vi "Main UI (ext control).vi"(0 "Serial port":refnum<visa-resource-name>="COM1", 1 "Command":T2, 5 "Data rate (Hz)":dbl=100.0, 7 "Max. num. sensors (override)":u8=64 max=64, 9 "Wait for HW trigger":bool, 11 "Finite samples":bool=TRUE, 12 "N samples":u32=1000, 14 "Error in":errorcluster) -> (4 "P data (mode 0)":T8[](array[typedef]), 15 "Error out":errorcluster)   [LabVIEW 2015]
doc: "User interface for 64 pressure multiplexer system designed by Paul Nathan, 02/2016"
uses:
  Ctls/System status.ctl
  Ctls/Environmental state values.ctl
  Ctls/Inertial state values.ctl
  Ctls/AccelGyro constants.ctl
  Ctls/Pressure sensor constants.ctl
  Ctls/Cmd list.ctl
  Ctls/Data values, Mode 0 (for datalog).ctl
  Ctls/Cmd str.ctl
  Ctls/All state values (for datalog).ctl
  Ctls/Data values, Mode 1 (for datalog).ctl
  Globals/PressureMultiplexer global.vi
panel:
  in  "Main tabs":T1(tab)
  in  "Env. period (ms)":i32=1000 min=0
  out "ACK 8":bool caption="ACK"
  out "ACK 7":bool caption="ACK"
  out "ACK 6":bool caption="ACK"
  out "AccelGyro constants":T3={"gyrRange"=125.0, "accRange"=2.0, "gx offset"=0.0, "gy offset"=0.0, "gz offset"=0.0, "ax offset"=0.0, "ay offset"=0.0, "az offset"=0.0, "axyz scale"=1.0} {"axyz scale" format="%#_4f"; "az offset" format="%#_4f"; "ay offset" format="%#_4f"; "ax offset" format="%#_4f"; "gz offset" format="%#_4f"; "gy offset" format="%#_4f"; "gx offset" format="%#_4f"; "gyrRange" format="%#_4f"; "accRange" format="%#_4f"}
  out "Faulty sensors":i32[](array[numeric])
  out "ACK 5":bool caption="ACK"
  out "Active sensors":i32[](array[numeric])
  out "ACK 4":bool caption="ACK"
  in  "Gyro. rate (Hz)":u8(ring) items=["6.25", "12.5", "25", "50", "100", "200", "400", "800", "1600", "3200"]
  in  "Gyro. range (dps)":u8(ring) items=["+/- 125", "+/- 250", "+/- 500", "+/- 1000", "+/- 2000"]
  in  "Accel. rate (Hz)":u8(ring)=1 items=["3.125", "6.25", "12.5", "25", "50", "100", "200", "400", "800", "1600"]
  in  "Accel. range (g)":u8(ring) items=["+/- 2", "+/- 4", "+/- 8", "+/- 16"]
  out "Inertial state values":T4 {"w_z (dps)" format="%#_4f"; "a_y (g)" format="%#_4f"; "a_z (g)" format="%#_4f"; "w_y (dps)" format="%#_4f"; "a_x (g)" format="%#_4f"; "Sensor temp. (degC)" format="%#.2f"; "w_x (dps)" format="%#_4f"}
  out "Environmental state values":T5 {"Dew point (degC)" format="%#.2f"; "Density (kg/m^3)" format="%#.3f"; "Pressure alt. (m)" format="%#.2f"; "Density alt. (m)" format="%#.2f"; "Rel. Humidity (%)" format="%#.2f"; "P_atmos (Pa)" format="%#_6f"; "Sensor temp. (degC)" format="%#.2f"; "Thermistor (degC)" format="%#.2f"}
  out "System status":T6
  out "ACK 3":bool caption="ACK"
  out "ACK 1":bool caption="ACK"
  in  "Data mode":u8(ring) items=["P", "P & T"]
  out "ACK 2":bool caption="ACK"
  out "Main Power":bool
  out "L_data (bytes)":u16
  out "Serial no.":u16 format="%04x"
  out "Active pressure sensor constants":T7[](array[typedef])
  out "Streaming":bool
  out "Clock drift":bool
  in  "Display rate (Hz)":dbl=100.0 min=0.0
  out "Sensor temperatures time trace (Mode \"P & T\" only)":sgl[][](graph)
  out "Pressures time trace":sgl[][](graph)
  in  "Stop streaming":bool
  out "Stale samples flag":u8[][](graph)
  out "Samples acquired":u32
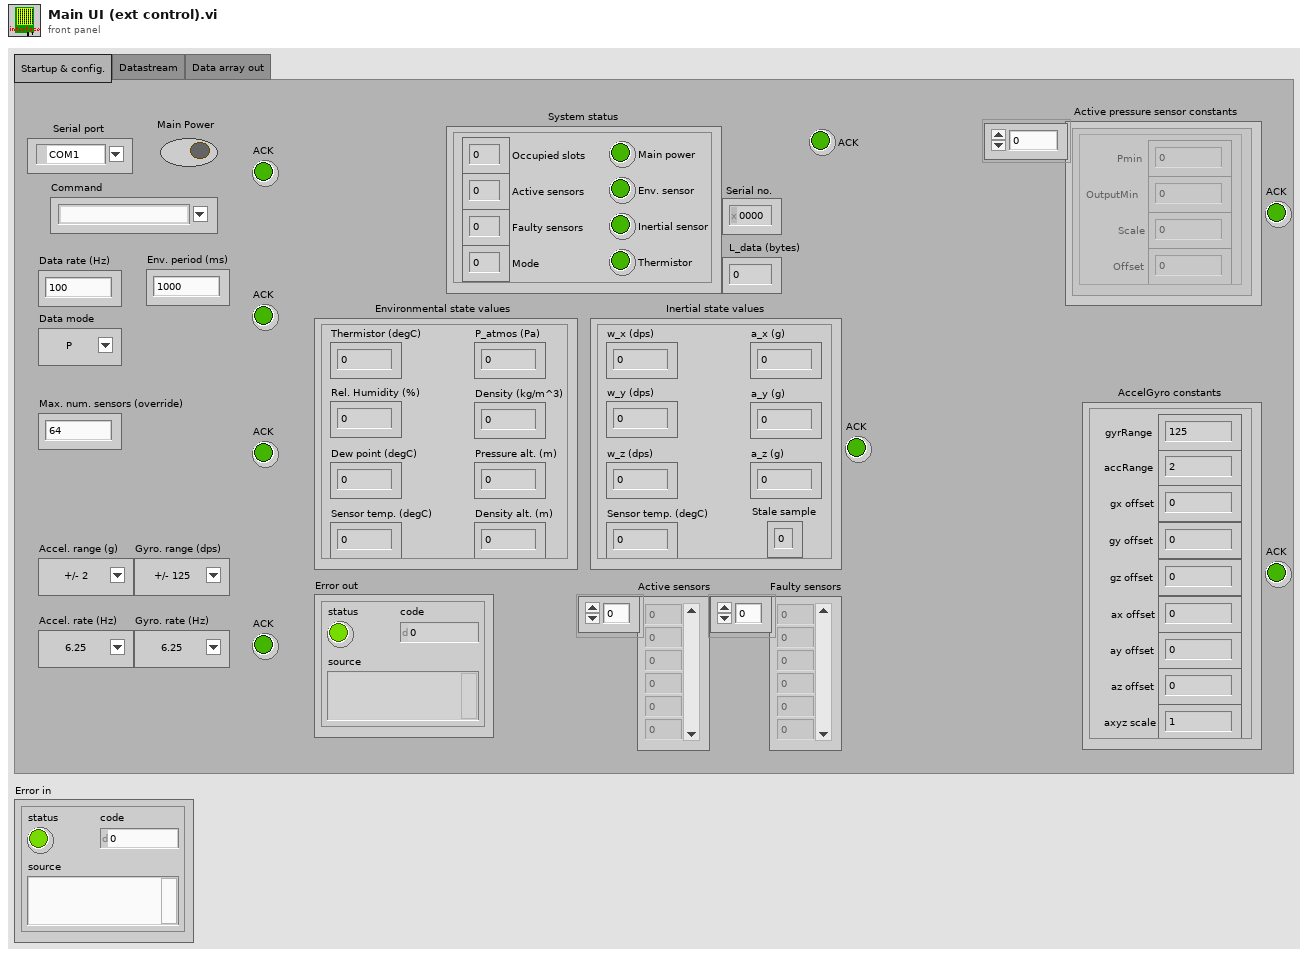
[diagram p1: front panel]
types:
  T1 = enum32{"Startup & config.", "Datastream", "Data array out"}
  T2 = typedef "Cmd list.ctl" = string
  T3 = typedef "AccelGyro constants.ctl" = cluster{"gyrRange":sgl, "accRange":sgl, "gx offset":sgl, "gy offset":sgl, "gz offset":sgl, "ax offset":sgl, "ay offset":sgl, "az offset":sgl, "axyz scale":sgl}
  T4 = typedef "Inertial state values.ctl" = cluster{"w_x (dps)":sgl, "w_y (dps)":sgl, "w_z (dps)":sgl, "a_x (g)":sgl, "a_y (g)":sgl, "a_z (g)":sgl, "Stale sample":u8, "Sensor temp. (degC)":sgl}
  T5 = typedef "Environmental state values.ctl" = cluster{"Thermistor (degC)":sgl, "Sensor temp. (degC)":sgl, "P_atmos (Pa)":sgl, "Rel. Humidity (%)":sgl, "Density (kg/m^3)":sgl, "Dew point (degC)":sgl, "Pressure alt. (m)":sgl, "Density alt. (m)":sgl}
  T6 = typedef "System status.ctl" = cluster{"Main power":bool, "Occupied slots":u8, "Active sensors":u8, "Faulty sensors":u8, "Env. sensor":bool, "Inertial sensor":bool, "Thermistor":bool, "Mode":u8}
  T7 = typedef "Pressure sensor constants.ctl" = cluster{"Pmin":sgl, "OutputMin":sgl, "Scale":sgl, "Offset":sgl}
  T8 = typedef "Data values, Mode 0 (for datalog).ctl" = cluster{"Time Stamp":timestamp, "dt (us)":sgl, "dt_warn":u8, "Pressures":sgl[], "Statuses":u8[]}
  T9 = typedef "All state values (for datalog).ctl" = cluster{"Time Stamp":timestamp, "dt (ms)":i32, "Environmental state values":T5, "Inertial state values":T4}
  T10 = typedef "Cmd str.ctl" = string
  T11 = typedef "Data values, Mode 1 (for datalog).ctl" = cluster{"Time Stamp":timestamp, "dt (us)":sgl, "dt_warn":u8, "Pressures":sgl[], "Die temps.":sgl[], "Statuses":u8[]}
  T12 = enum8{"Enabled", "Disabled", "Disabled and Grayed Out"}
  T13 = typedef "EEPROM page.ctl" = cluster{"Pmin (Pa)":sgl, "Pmax (Pa)":sgl, "maxCount":u16, "minCount":u16, "Poffset (Pa)":sgl}
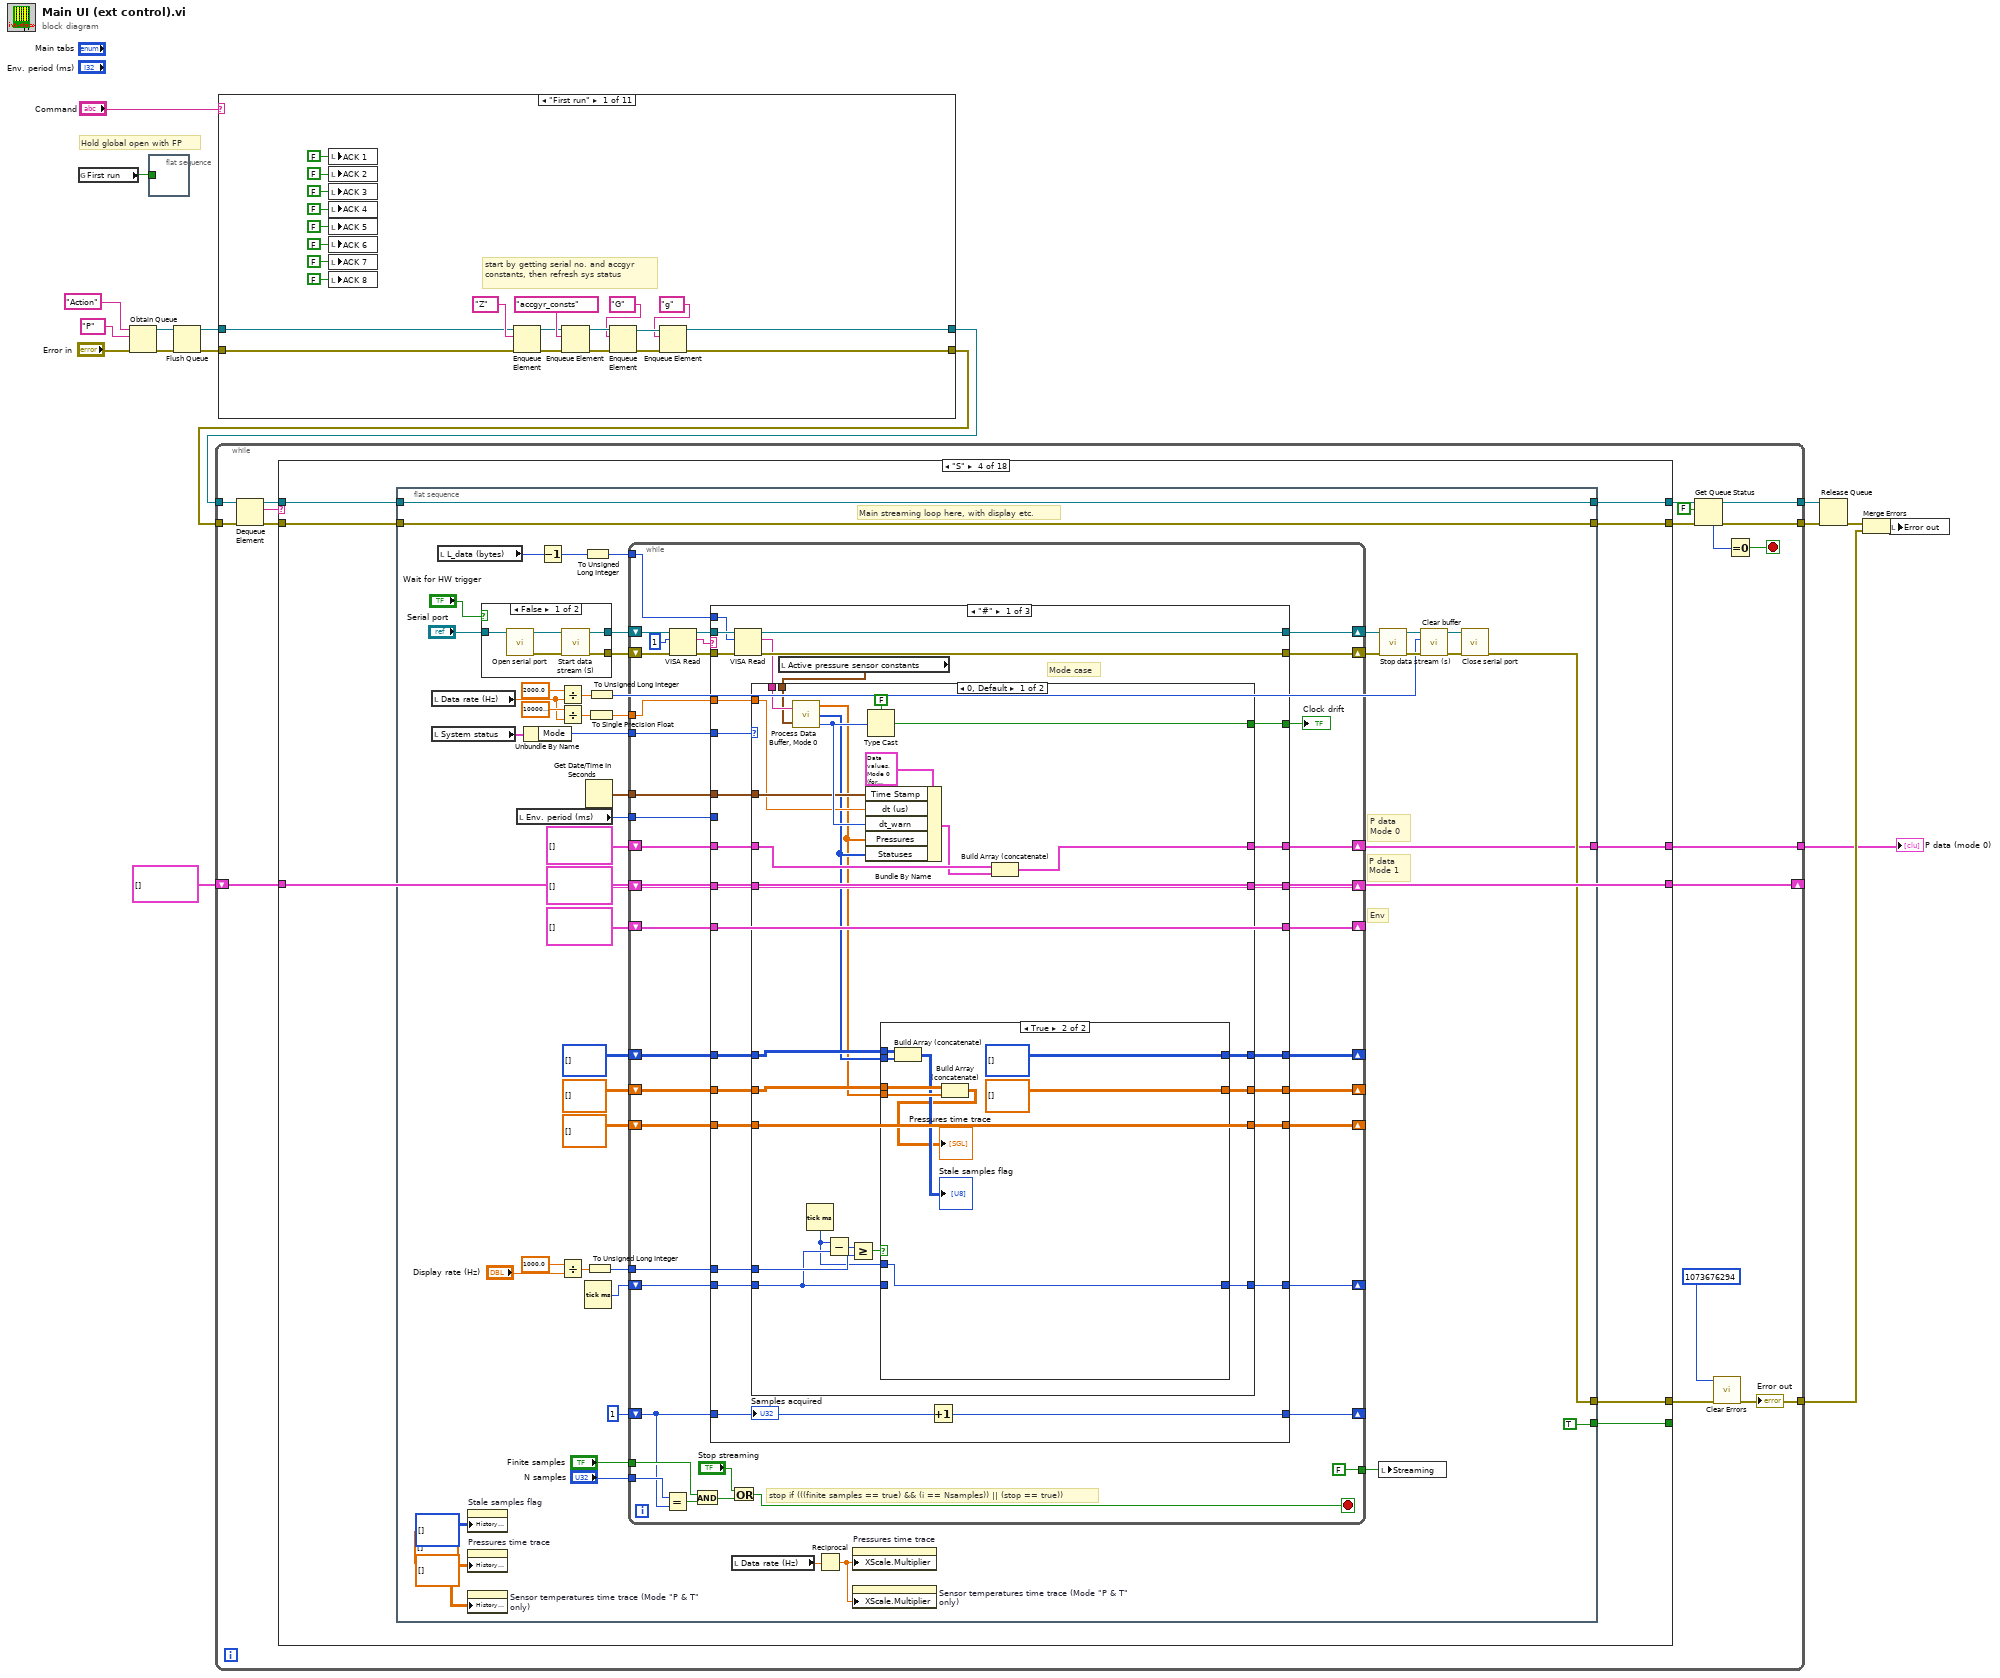
[diagram p0: block diagram]
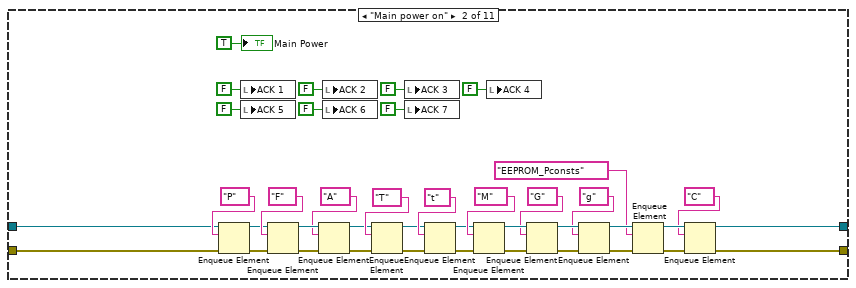
[diagram p2: hidden frame]
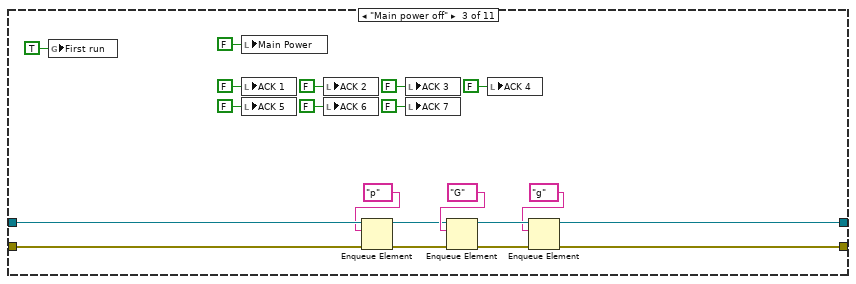
[diagram p3: hidden frame]
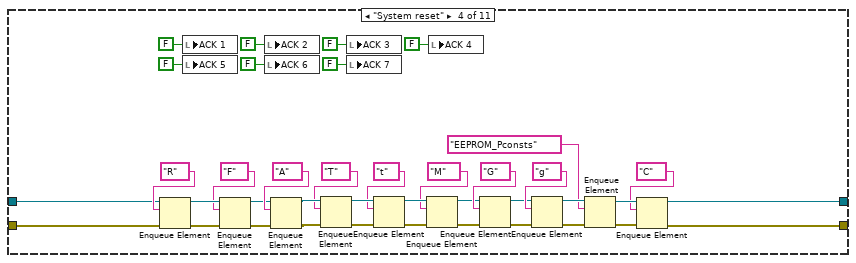
[diagram p4: hidden frame]
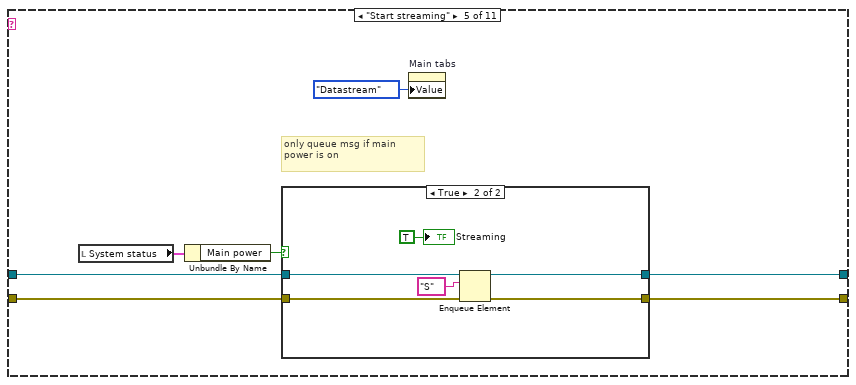
[diagram p5: hidden frame]
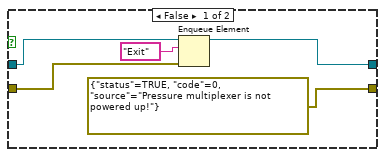
[diagram p6: hidden frame]
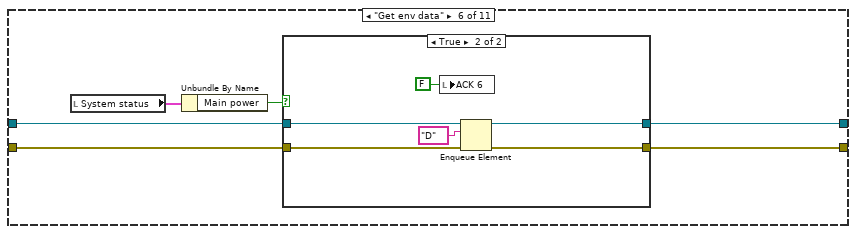
[diagram p7: hidden frame]
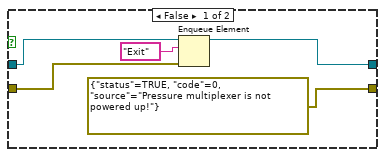
[diagram p8: hidden frame]
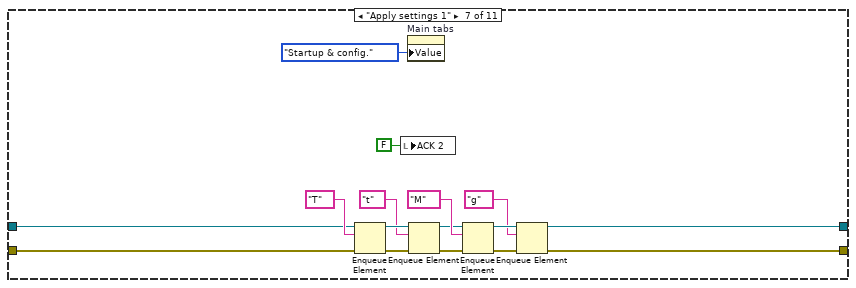
[diagram p9: hidden frame]
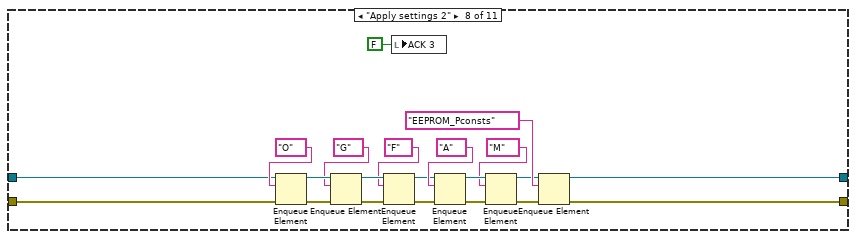
[diagram p10: hidden frame]
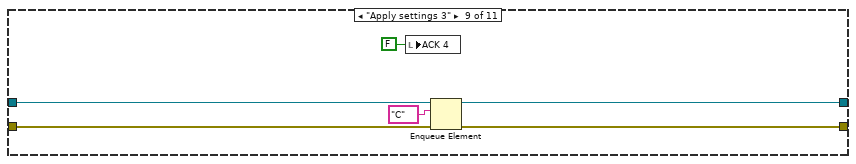
[diagram p11: hidden frame]
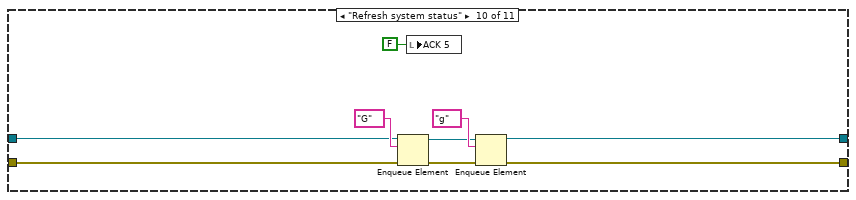
[diagram p12: hidden frame]
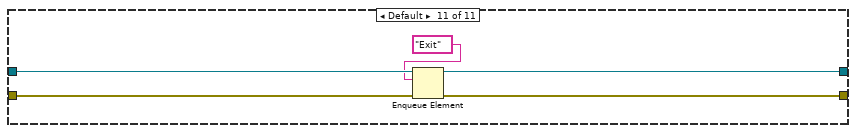
[diagram p13: hidden frame]
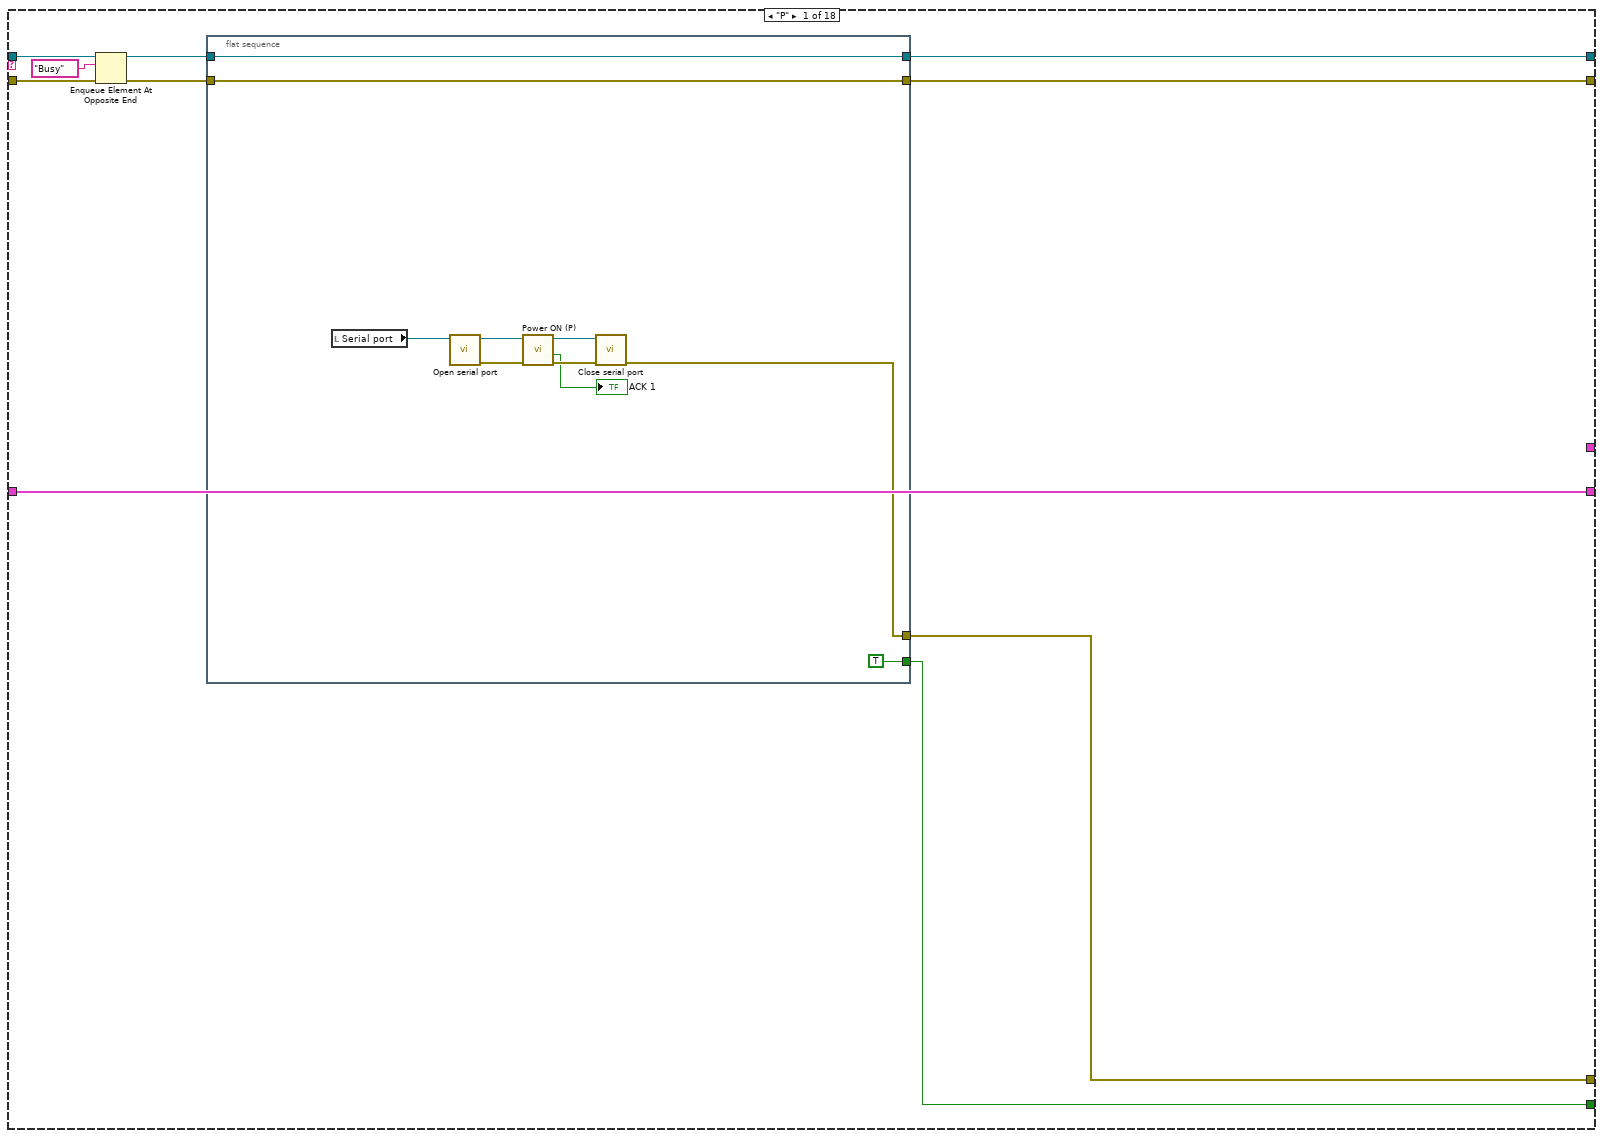
[diagram p14: hidden frame]
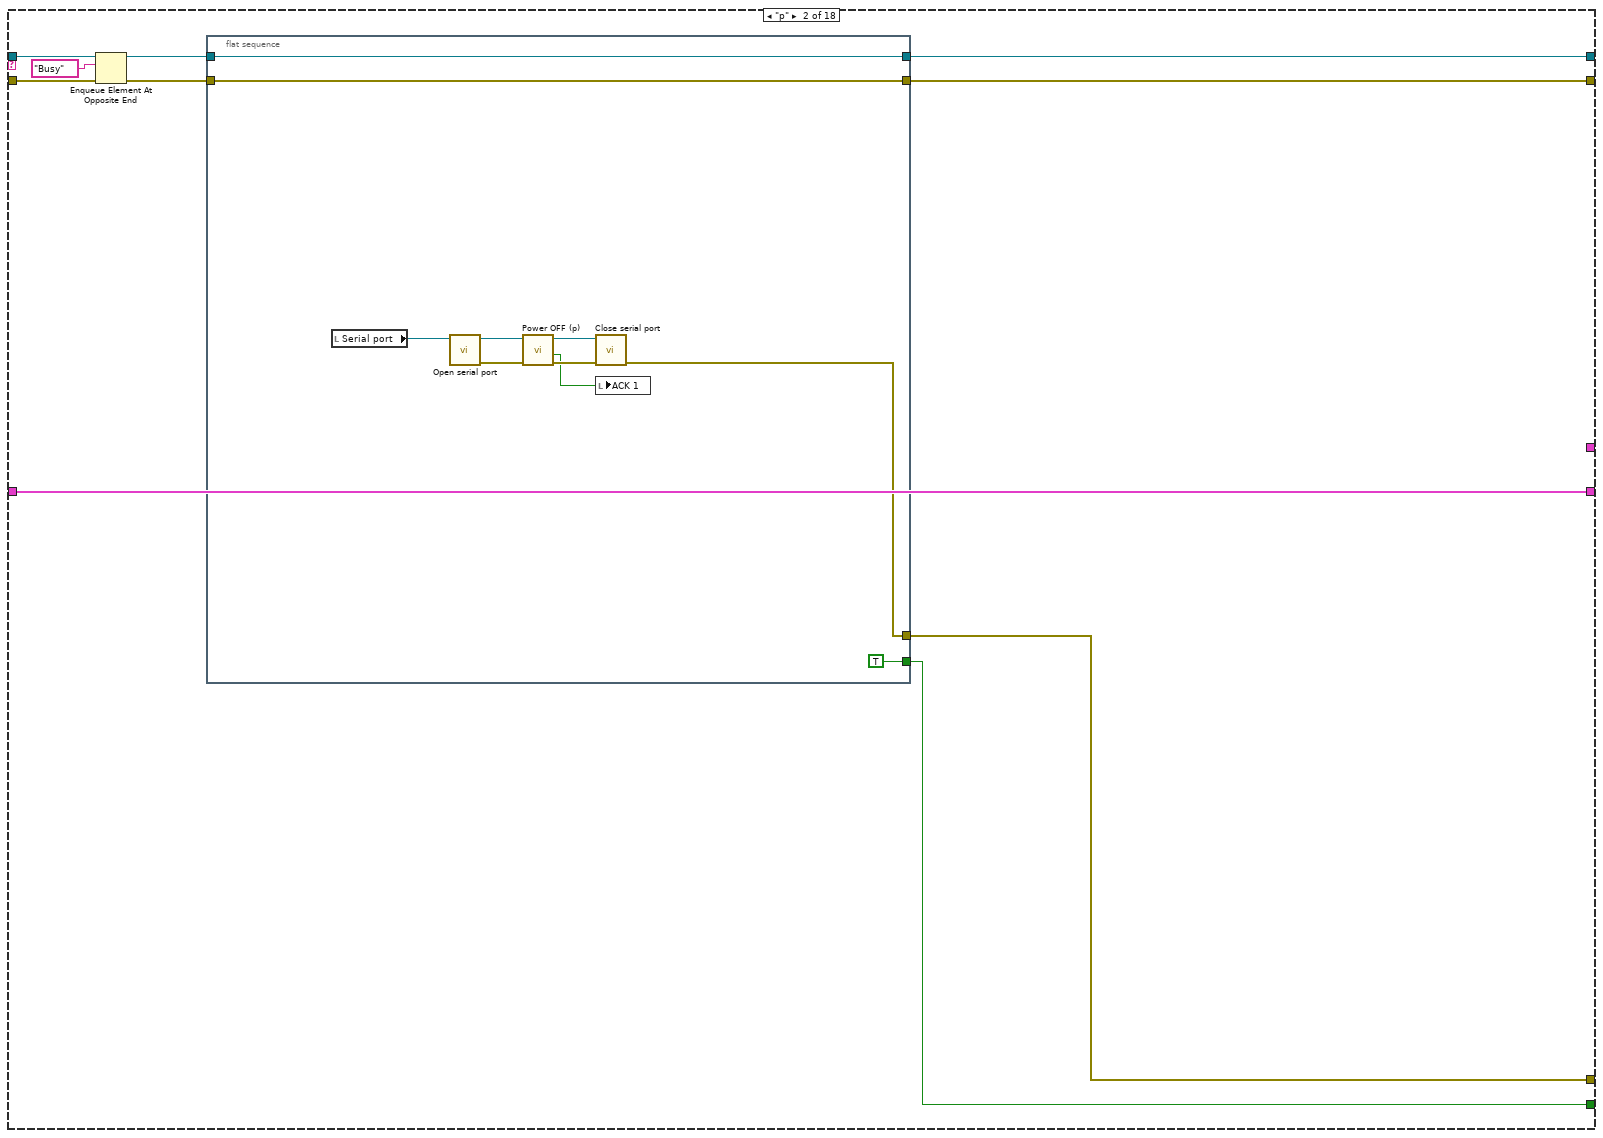
[diagram p15: hidden frame]
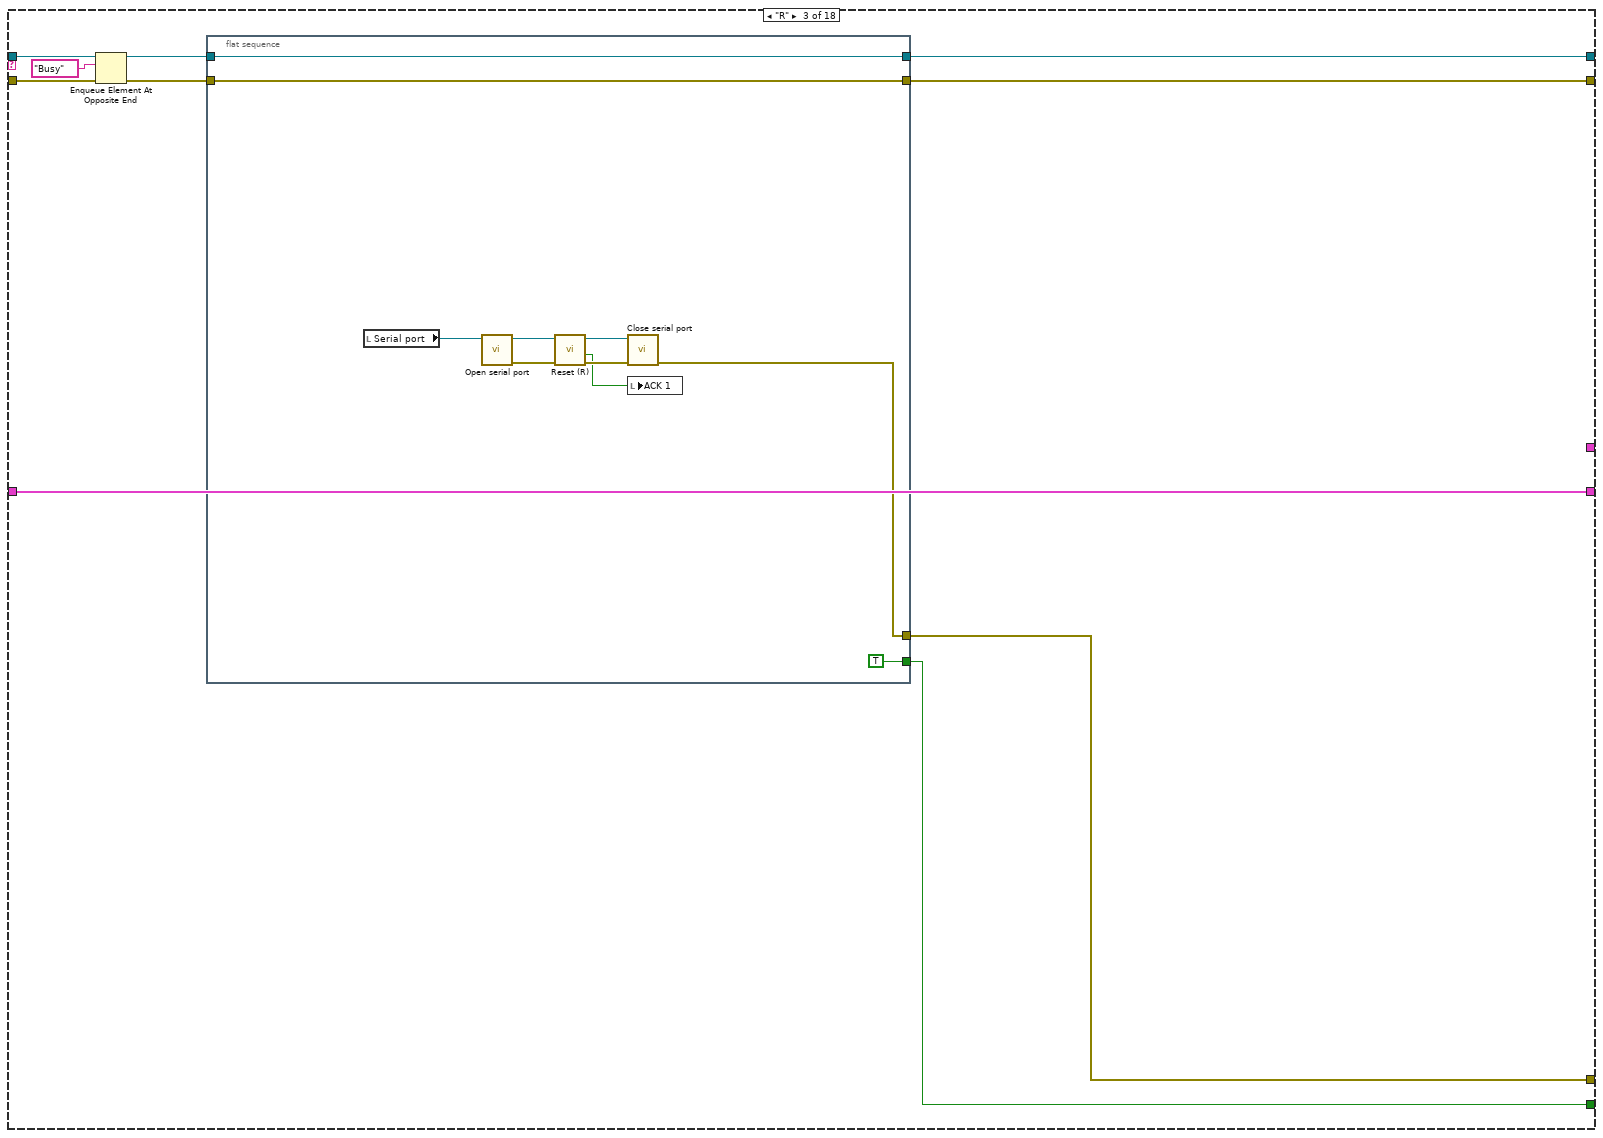
[diagram p16: hidden frame]
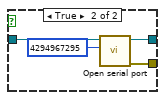
[diagram p17: hidden frame]
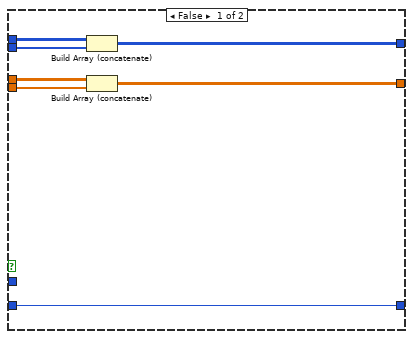
[diagram p18: hidden frame]
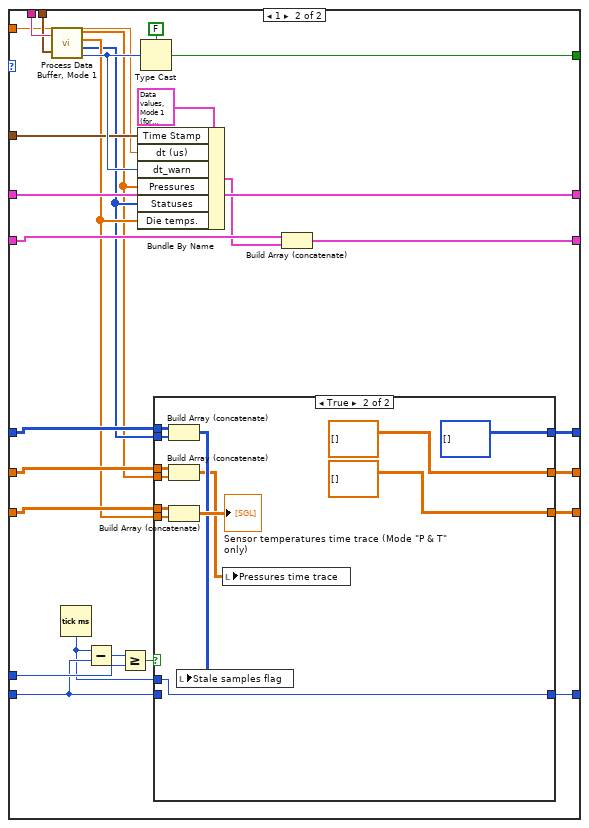
[diagram p19: hidden frame]
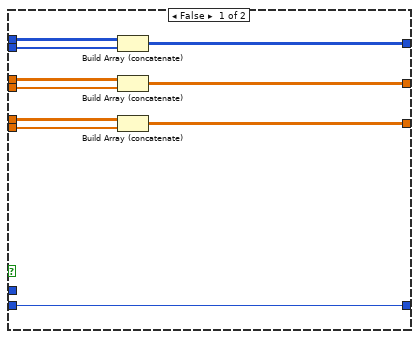
[diagram p20: hidden frame]
diagram:
  # "Hold global open with FP"
  n1 = global read "PressureMultiplexer global.vi" "First run"() -> (w1:bool)
  n2 = Obtain Queue(name (unnamed)="Action", element data type=T10 "P" ("Cmd"), error in (no error)="Error in") -> (queue out=w17:refnum<queue>, error out=w16:errorcluster)  [unwired: 2 in, 1 out]
  n3 = flat-sequence {
    tunnel: w1 -> [_]
    frame #0 {
    }
  }
  n4 = Flush Queue(queue=w17, error in (no error)=w16) -> (queue out=w5:refnum<queue>, error out=w4:errorcluster)  [unwired: 1 out]
  n5 = case shown="\"First run\"" "Command" {
    tunnel: [w28 w51 w92 w109 w141 w160 w178 w193 w214 w219 w227] -> w8
    tunnel: w4 -> [w29 w78 w99 w110 w144 w161 w179 w194 w215 w222 w231]
    tunnel: w5 -> [w30 w79 w100 w111 w143 w162 w180 w195 w216 w221 w230]
    tunnel: [w27 w50 w91 w108 w142 w159 w177 w192 w213 w220 w228] -> w7
    frame "First run" {
      # "start by getting serial no. and accgyr constants, then refresh sys status"
      n6 = local write "ACK 1"(FALSE ("ACK 8")) -> ()
      n7 = local write "ACK 2"(FALSE ("ACK 6")) -> ()
      n8 = local write "ACK 3"(FALSE ("ACK 8")) -> ()
      n9 = local write "ACK 4"(FALSE ("Done")) -> ()
      n10 = local write "ACK 5"(FALSE ("ACK 8")) -> ()
      n11 = local write "ACK 6"(FALSE ("ACK 6")) -> ()
      n12 = local write "ACK 7"(FALSE ("ACK 6")) -> ()
      n13 = local write "ACK 8"(FALSE ("ACK 8")) -> ()
      n14 = Enqueue Element(queue=w30, element=T10 "Z", error in (no error)=w29) -> (queue out=w32:refnum<queue>, error out=w33:errorcluster)  [unwired: 1 in, 1 out]
      n15 = Enqueue Element(queue=w32, element=T10 "accgyr_consts", error in (no error)=w33) -> (queue out=w39:refnum<queue>, error out=w40:errorcluster)  [unwired: 1 in, 1 out]
      n16 = Enqueue Element(queue=w39, element=T10 "G" ("Cmd"), error in (no error)=w40) -> (queue out=w37:refnum<queue>, error out=w36:errorcluster)  [unwired: 1 in, 1 out]
      n17 = Enqueue Element(queue=w37, element=T10 "g" ("Cmd"), error in (no error)=w36) -> (queue out=w27:refnum<queue>, error out=w28:errorcluster)  [unwired: 1 in, 1 out]
    }
    frame "Main power on" {
      n18 = Enqueue Element(queue=w79, element=T10 "P" ("Cmd"), error in (no error)=w78) -> (queue out=w72:refnum<queue>, error out=w71:errorcluster)  [unwired: 1 in, 1 out]
      n19 = local write "ACK 1"(FALSE ("ACK 1")) -> ()
      n20 = local write "ACK 5"(FALSE ("ACK 8")) -> ()
      n21 = Enqueue Element(queue=w72, element=T10 "F" ("Cmd"), error in (no error)=w71) -> (queue out=w76:refnum<queue>, error out=w77:errorcluster)  [unwired: 1 in, 1 out]
      n22 = Enqueue Element(queue=w76, element=T10 "A" ("Cmd"), error in (no error)=w77) -> (queue out=w57:refnum<queue>, error out=w56:errorcluster)  [unwired: 1 in, 1 out]
      n23 = local write "ACK 2"(FALSE ("ACK 6")) -> ()
      n24 = local write "ACK 6"(FALSE ("ACK 6")) -> ()
      n25 = Enqueue Element(queue=w57, element=T10 "T" ("Cmd"), error in (no error)=w56) -> (queue out=w59:refnum<queue>, error out=w58:errorcluster)  [unwired: 1 in, 1 out]
      n26 = local write "ACK 3"(FALSE ("ACK 8")) -> ()
      n27 = local write "ACK 7"(FALSE ("ACK 6")) -> ()
      n28 = Enqueue Element(queue=w59, element=T10 "t" ("Cmd"), error in (no error)=w58) -> (queue out=w54:refnum<queue>, error out=w55:errorcluster)  [unwired: 1 in, 1 out]
      n29 = Enqueue Element(queue=w54, element=T10 "M" ("Cmd"), error in (no error)=w55) -> (queue out=w68:refnum<queue>, error out=w67:errorcluster)  [unwired: 1 in, 1 out]
      n30 = local write "ACK 4"(FALSE ("Done")) -> ()
      n31 = Enqueue Element(queue=w68, element=T10 "G" ("Cmd"), error in (no error)=w67) -> (queue out=w69:refnum<queue>, error out=w70:errorcluster)  [unwired: 1 in, 1 out]
      n32 = Enqueue Element(queue=w69, element=T10 "g" ("Cmd"), error in (no error)=w70) -> (queue out=w64:refnum<queue>, error out=w63:errorcluster)  [unwired: 1 in, 1 out]
      n33 = Enqueue Element(queue=w64, element=T10 "EEPROM_Pconsts" ("Cmd"), error in (no error)=w63) -> (queue out=w53:refnum<queue>, error out=w52:errorcluster)  [unwired: 1 in, 1 out]
      n34 = Enqueue Element(queue=w53, element=T10 "C" ("Cmd"), error in (no error)=w52) -> (queue out=w50:refnum<queue>, error out=w51:errorcluster)  [unwired: 1 in, 1 out]
      "Main Power" <- TRUE ("Main Power")
    }
    frame "Main power off" {
      n35 = global write "PressureMultiplexer global.vi" "First run"(TRUE ("First run")) -> ()
      n36 = local write "Main Power"(FALSE ("Main Power")) -> ()
      n37 = local write "ACK 1"(FALSE ("ACK 1")) -> ()
      n38 = local write "ACK 5"(FALSE ("ACK 8")) -> ()
      n39 = local write "ACK 2"(FALSE ("ACK 6")) -> ()
      n40 = local write "ACK 6"(FALSE ("ACK 6")) -> ()
      n41 = Enqueue Element(queue=w100, element=T10 "p" ("Cmd"), error in (no error)=w99) -> (queue out=w96:refnum<queue>, error out=w95:errorcluster)  [unwired: 1 in, 1 out]
      n42 = local write "ACK 3"(FALSE ("ACK 8")) -> ()
      n43 = local write "ACK 7"(FALSE ("ACK 6")) -> ()
      n44 = Enqueue Element(queue=w96, element=T10 "G" ("Cmd"), error in (no error)=w95) -> (queue out=w94:refnum<queue>, error out=w93:errorcluster)  [unwired: 1 in, 1 out]
      n45 = local write "ACK 4"(FALSE ("Done")) -> ()
      n46 = Enqueue Element(queue=w94, element=T10 "g" ("Cmd"), error in (no error)=w93) -> (queue out=w91:refnum<queue>, error out=w92:errorcluster)  [unwired: 1 in, 1 out]
    }
    frame "System reset" {
      n47 = Enqueue Element(queue=w111, element=T10 "R" ("Cmd"), error in (no error)=w110) -> (queue out=w123:refnum<queue>, error out=w124:errorcluster)  [unwired: 1 in, 1 out]
      n48 = local write "ACK 1"(FALSE ("ACK 1")) -> ()
      n49 = local write "ACK 5"(FALSE ("ACK 8")) -> ()
      n50 = Enqueue Element(queue=w123, element=T10 "F" ("Cmd"), error in (no error)=w124) -> (queue out=w115:refnum<queue>, error out=w125:errorcluster)  [unwired: 1 in, 1 out]
      n51 = local write "ACK 2"(FALSE ("ACK 6")) -> ()
      n52 = local write "ACK 6"(FALSE ("ACK 6")) -> ()
      n53 = Enqueue Element(queue=w115, element=T10 "A" ("Cmd"), error in (no error)=w125) -> (queue out=w133:refnum<queue>, error out=w134:errorcluster)  [unwired: 1 in, 1 out]
      n54 = Enqueue Element(queue=w133, element=T10 "T" ("Cmd"), error in (no error)=w134) -> (queue out=w131:refnum<queue>, error out=w132:errorcluster)  [unwired: 1 in, 1 out]
      n55 = local write "ACK 3"(FALSE ("ACK 8")) -> ()
      n56 = local write "ACK 7"(FALSE ("ACK 6")) -> ()
      n57 = Enqueue Element(queue=w131, element=T10 "t" ("Cmd"), error in (no error)=w132) -> (queue out=w135:refnum<queue>, error out=w136:errorcluster)  [unwired: 1 in, 1 out]
      n58 = Enqueue Element(queue=w135, element=T10 "M" ("Cmd"), error in (no error)=w136) -> (queue out=w119:refnum<queue>, error out=w126:errorcluster)  [unwired: 1 in, 1 out]
      n59 = local write "ACK 4"(FALSE ("Done")) -> ()
      n60 = Enqueue Element(queue=w119, element=T10 "G" ("Cmd"), error in (no error)=w126) -> (queue out=w118:refnum<queue>, error out=w127:errorcluster)  [unwired: 1 in, 1 out]
      n61 = Enqueue Element(queue=w118, element=T10 "g" ("Cmd"), error in (no error)=w127) -> (queue out=w122:refnum<queue>, error out=w128:errorcluster)  [unwired: 1 in, 1 out]
      n62 = Enqueue Element(queue=w122, element=T10 "EEPROM_Pconsts" ("Cmd"), error in (no error)=w128) -> (queue out=w138:refnum<queue>, error out=w139:errorcluster)  [unwired: 1 in, 1 out]
      n63 = Enqueue Element(queue=w138, element=T10 "C" ("Cmd"), error in (no error)=w139) -> (queue out=w108:refnum<queue>, error out=w109:errorcluster)  [unwired: 1 in, 1 out]
    }
    frame "Start streaming" {
      # "only queue msg if main power is on"
      n64 = local read "System status"() -> (w146:T6)
      n65 = Unbundle By Name(w146) -> ("Main power"=w145:bool)
      n66 = case shown="True" w145 {
        tunnel: w143 -> [w149 w156]
        tunnel: w144 -> [w147 w155]
        tunnel: [w148 w153] -> w142
        tunnel: [errorcluster {"status"=TRUE, "code"=0, "source"="Pressure multiplexer is not powered up!"} ("error out") w154] -> w141
        frame False {
          n67 = Enqueue Element(queue=w149, element=T10 "Exit" ("Cmd"), error in (no error)=w147) -> (queue out=w148:refnum<queue>)  [unwired: 1 in, 2 out]
        }
        frame True {
          n68 = Enqueue Element(queue=w156, element=T10 "S" ("Cmd"), error in (no error)=w155) -> (queue out=w153:refnum<queue>, error out=w154:errorcluster)  [unwired: 1 in, 1 out]
          "Streaming" <- TRUE ("Streaming")
        }
      }
      n69 = property on="Main tabs" class="TabCtl (strict)"("Value"=T1."Datastream" ("Main tabs")) -> ()  [unwired: 2 in, 2 out]
    }
    frame "Get env data" {
      n70 = local read "System status"() -> (w163:T6)
      n71 = Unbundle By Name(w163) -> ("Main power"=w158:bool)
      n72 = case shown="True" w158 {
        tunnel: w162 -> [w166 w173]
        tunnel: w161 -> [w164 w172]
        tunnel: [w165 w170] -> w159
        tunnel: [errorcluster {"status"=TRUE, "code"=0, "source"="Pressure multiplexer is not powered up!"} ("error out") w171] -> w160
        frame False {
          n73 = Enqueue Element(queue=w166, element=T10 "Exit" ("Cmd"), error in (no error)=w164) -> (queue out=w165:refnum<queue>)  [unwired: 1 in, 2 out]
        }
        frame True {
          n74 = local write "ACK 6"(FALSE ("ACK 6")) -> ()
          n75 = Enqueue Element(queue=w173, element=T10 "D" ("Cmd"), error in (no error)=w172) -> (queue out=w170:refnum<queue>, error out=w171:errorcluster)  [unwired: 1 in, 1 out]
        }
      }
    }
    frame "Apply settings 1" {
      n76 = Enqueue Element(queue=w180, element=T10 "T" ("Cmd"), error in (no error)=w179) -> (queue out=w183:refnum<queue>, error out=w184:errorcluster)  [unwired: 1 in, 1 out]
      n77 = local write "ACK 2"(FALSE ("ACK 6")) -> ()
      n78 = property on="Main tabs" class="TabCtl (strict)"("Value"=T1."Startup & config." ("Main tabs")) -> ()  [unwired: 2 in, 2 out]
      n79 = Enqueue Element(queue=w183, element=T10 "t" ("Cmd"), error in (no error)=w184) -> (queue out=w186:refnum<queue>, error out=w185:errorcluster)  [unwired: 1 in, 1 out]
      n80 = Enqueue Element(queue=w186, element=T10 "M" ("Cmd"), error in (no error)=w185) -> (queue out=w189:refnum<queue>, error out=w190:errorcluster)  [unwired: 1 in, 1 out]
      n81 = Enqueue Element(queue=w189, element=T10 "g" ("Cmd"), error in (no error)=w190) -> (queue out=w177:refnum<queue>, error out=w178:errorcluster)  [unwired: 1 in, 1 out]
    }
    frame "Apply settings 2" {
      n82 = Enqueue Element(queue=w195, element=T10 "O" ("Cmd"), error in (no error)=w194) -> (queue out=w198:refnum<queue>, error out=w199:errorcluster)  [unwired: 1 in, 1 out]
      n83 = Enqueue Element(queue=w198, element=T10 "G" ("Cmd"), error in (no error)=w199) -> (queue out=w210:refnum<queue>, error out=w211:errorcluster)  [unwired: 1 in, 1 out]
      n84 = Enqueue Element(queue=w210, element=T10 "F" ("Cmd"), error in (no error)=w211) -> (queue out=w206:refnum<queue>, error out=w205:errorcluster)  [unwired: 1 in, 1 out]
      n85 = local write "ACK 3"(FALSE ("ACK 8")) -> ()
      n86 = Enqueue Element(queue=w206, element=T10 "A" ("Cmd"), error in (no error)=w205) -> (queue out=w208:refnum<queue>, error out=w209:errorcluster)  [unwired: 1 in, 1 out]
      n87 = Enqueue Element(queue=w208, element=T10 "M" ("Cmd"), error in (no error)=w209) -> (queue out=w201:refnum<queue>, error out=w200:errorcluster)  [unwired: 1 in, 1 out]
      n88 = Enqueue Element(queue=w201, element=T10 "EEPROM_Pconsts" ("Cmd"), error in (no error)=w200) -> (queue out=w192:refnum<queue>, error out=w193:errorcluster)  [unwired: 1 in, 1 out]
    }
    frame "Apply settings 3" {
      n89 = local write "ACK 4"(FALSE ("Done")) -> ()
      n90 = Enqueue Element(queue=w216, element=T10 "C" ("Cmd"), error in (no error)=w215) -> (queue out=w213:refnum<queue>, error out=w214:errorcluster)  [unwired: 1 in, 1 out]
    }
    frame "Refresh system status" {
      n91 = Enqueue Element(queue=w221, element=T10 "G" ("Cmd"), error in (no error)=w222) -> (queue out=w224:refnum<queue>, error out=w225:errorcluster)  [unwired: 1 in, 1 out]
      n92 = local write "ACK 5"(FALSE ("ACK 8")) -> ()
      n93 = Enqueue Element(queue=w224, element=T10 "g" ("Cmd"), error in (no error)=w225) -> (queue out=w220:refnum<queue>, error out=w219:errorcluster)  [unwired: 1 in, 1 out]
    }
    frame Default {
      n94 = Enqueue Element(queue=w230, element=T10 "Exit" ("Cmd"), error in (no error)=w231) -> (queue out=w228:refnum<queue>, error out=w227:errorcluster)  [unwired: 1 in, 1 out]
    }
  }
  n95 = while {
    tunnel: w8 -> [w248]
    tunnel: w7 -> [w249]
    tunnel: [w236] -> w15
    shift-right: [w244] -> _
    shift-left: T9[] [] -> [w243]
    tunnel: [w240] -> w11
    tunnel: [w233] -> w9
    tunnel: [w232] -> w3
    stop <- w234 stop-if-true
    n96 = Dequeue Element(queue=w249, error in (no error)=w248) -> (queue out=w247:refnum<queue>, element=w245:T10, error out=w246:errorcluster)  [unwired: 1 in, 1 out]
    n97 = case shown="\"S\"" w245 {
      tunnel: w247 -> [w259 w279 w299 w317 w572 w592 w611 w630 w649 w672 w704 w721 w738 w772 w790 w819 w846 w863]
      tunnel: w246 -> [w258 w278 w298 w316 w571 w591 w610 w629 w648 w671 w703 w720 w737 w771 w789 w818 w845 w867]
      tunnel: [w254 w274 w294 w311 w569 w589 w608 w627 w646 w669 w701 w718 w735 w769 w787 w816 w843 w867] -> w238
      tunnel: [w253 w273 w293 w315 w568 w588 w607 w626 w645 w668 w700 w717 w734 w768 w786 w815 w842 FALSE] -> _
      tunnel: [w252 w272 w292 w314 w567 w587 w606 w625 w644 w667 w699 w716 w733 w767 w785 w814 w841 errorcluster {"status"=FALSE, "code"=0, "source"=""} ("Error out")] -> w241
      tunnel: [w250 w270 w290 w313 w566 w586 w605 w624 w643 w666 w698 w715 w732 w766 w784 w813 w840 w864] -> w244
      tunnel: w243 -> [w250 w270 w290 w313 w566 w586 w605 w624 w643 w666 w698 w715 w732 w766 w783 w813 w840 w864]
      tunnel: [w255 w275 w295 w312 w570 w590 w609 w628 w647 w670 w702 w719 w736 w770 w788 w817 w844 w863] -> w239
      tunnel: [_ _ _ w310 _ _ _ _ _ _ _ _ _ _ _ _ _ _] -> w232
      frame "P" {
        n98 = Enqueue Element At Opposite End(queue=w259, element=T10 "Busy" ("Cmd"), error in (no error)=w258) -> (queue out=w257:refnum<queue>, error out=w256:errorcluster)  [unwired: 1 in, 1 out]
        n99 = flat-sequence {
          tunnel: w257 -> [w269]
          tunnel: w256 -> [w268]
          tunnel: [w269] -> w255
          tunnel: [w268] -> w254
          tunnel: [TRUE] -> w253
          tunnel: [w262] -> w252
          frame #0 {
            n100 = local read "Serial port"() -> (w261:refnum<visa-resource-name>)
            n101 = call "Open serial port.vi"("VISA resource name"=w261) -> ("Error out"=w265:errorcluster, "VISA resource name out"=w266:refnum<visa-resource-name>)  [unwired: 9 in]
            n102 = call "Power ON (P).vi"("Error In"=w265, "VISA resource name in"=w266) -> ("Error out"=w264:errorcluster, "ACK"=→"ACK 1":bool, "VISA resource name out"=w263:refnum<visa-resource-name>)  [unwired: 7 in]
            n103 = call "Close serial port.vi"("Error in"=w264, "VISA resource name"=w263) -> ("Error out"=w262:errorcluster)  [unwired: 9 in]
          }
        }
      }
      frame "p" {
        n104 = Enqueue Element At Opposite End(queue=w279, element=T10 "Busy" ("Cmd"), error in (no error)=w278) -> (queue out=w277:refnum<queue>, error out=w276:errorcluster)  [unwired: 1 in, 1 out]
        n105 = flat-sequence {
          tunnel: w277 -> [w289]
          tunnel: w276 -> [w288]
          tunnel: [w289] -> w275
          tunnel: [w288] -> w274
          tunnel: [TRUE] -> w273
          tunnel: [w282] -> w272
          frame #0 {
            n106 = local read "Serial port"() -> (w280:refnum<visa-resource-name>)
            n107 = call "Open serial port.vi"("VISA resource name"=w280) -> ("Error out"=w285:errorcluster, "VISA resource name out"=w286:refnum<visa-resource-name>)  [unwired: 9 in]
            n108 = call "Power OFF (p).vi"("Error In"=w285, "VISA resource name in"=w286) -> ("Error out"=w284:errorcluster, "ACK"=w281:bool, "VISA resource name out"=w283:refnum<visa-resource-name>)  [unwired: 7 in]
            n109 = call "Close serial port.vi"("Error in"=w284, "VISA resource name"=w283) -> ("Error out"=w282:errorcluster)  [unwired: 9 in]
            n110 = local write "ACK 1"(w281) -> ()
          }
        }
      }
      frame "R" {
        n111 = Enqueue Element At Opposite End(queue=w299, element=T10 "Busy" ("Cmd"), error in (no error)=w298) -> (queue out=w297:refnum<queue>, error out=w296:errorcluster)  [unwired: 1 in, 1 out]
        n112 = flat-sequence {
          tunnel: w297 -> [w309]
          tunnel: w296 -> [w308]
          tunnel: [w309] -> w295
          tunnel: [w308] -> w294
          tunnel: [TRUE] -> w293
          tunnel: [w304] -> w292
          frame #0 {
            n113 = local read "Serial port"() -> (w302:refnum<visa-resource-name>)
            n114 = call "Open serial port.vi"("VISA resource name"=w302) -> ("Error out"=w300:errorcluster, "VISA resource name out"=w301:refnum<visa-resource-name>)  [unwired: 9 in]
            n115 = call "Reset (R).vi"("Error In"=w300, "VISA resource name in"=w301) -> ("Error out"=w306:errorcluster, "ACK"=w303:bool, "VISA resource name out"=w305:refnum<visa-resource-name>)  [unwired: 7 in]
            n116 = call "Close serial port.vi"("Error in"=w306, "VISA resource name"=w305) -> ("Error out"=w304:errorcluster)  [unwired: 9 in]
            n117 = local write "ACK 1"(w303) -> ()
          }
        }
      }
      frame "S" {
        n118 = flat-sequence {
          tunnel: w317 -> [w366]
          tunnel: w316 -> [w365]
          tunnel: [w366] -> w312
          tunnel: [w365] -> w311
          tunnel: [TRUE] -> w315
          tunnel: [w320] -> w314
          tunnel: [w319] -> w310
          frame #0 {
            # "Env"
            # "P data Mode 1"
            # "P data Mode 0"
            # "Main streaming loop here, with display etc."
            n119 = local read "Data rate (Hz)"() -> (w340:dbl)
            n120 = local read "System status"() -> (w337:T6)
            n121 = local read "L_data (bytes)"() -> (w344:u16)
            n122 = property on="Stale samples flag" class="WFChart (strict)"("History Data"=u8[][] []) -> ()  [unwired: 2 in, 2 out]
            n123 = property on="Pressures time trace" class="WFChart (strict)"("History Data"=sgl[][] []) -> ()  [unwired: 2 in, 2 out]
            n124 = property on="Sensor temperatures time trace (Mode \"P & T\" only)" class="WFChart (strict)"("History Data"=sgl[][] []) -> ()  [unwired: 2 in, 2 out]
            n125 = case shown="False" "Wait for HW trigger" {
              tunnel: [w369 w373] -> w363
              tunnel: [w368 w374] -> w362
              tunnel: "Serial port" -> [w367 w375]
              frame False {
                n126 = call "Open serial port.vi"("VISA resource name"=w367) -> ("Error out"=w370:errorcluster, "VISA resource name out"=w371:refnum<visa-resource-name>)  [unwired: 9 in]
                n127 = call "Start data stream (S).vi"("VISA resource name in"=w371, "Error In"=w370) -> ("VISA resource name out"=w368:refnum<visa-resource-name>, "Error out"=w369:errorcluster)  [unwired: 7 in]
              }
              frame True {
                n128 = call "Open serial port.vi"("timeout (ms)"=u32 4294967295, "VISA resource name"=w375) -> ("Error out"=w373:errorcluster, "VISA resource name out"=w374:refnum<visa-resource-name>)  [unwired: 8 in]
              }
            }
            n129 = local read "Env. period (ms)"() -> (w342:i32)
            n130 = Unbundle By Name(w337) -> ("Mode"=w326:u8)
            n131 = Decrement(x=w344) -> (x-1=w327:u16)
            n132 = Divide(x=2000.0 ("y"), y=w340) -> (x/y=w356:dbl)
            n133 = Divide(x=1000000.0 ("y"), y=w340) -> (x/y=w339:dbl)
            n134 = Divide(x=1000.0, y="Display rate (Hz)") -> (x/y=w351:dbl)
            n135 = To Unsigned Long Integer(number=w327) -> (unsigned 32bit integer=w343:u32)
            n136 = Tick Count (ms)() -> (millisecond timer value=w328:u32)
            n137 = Get Date/Time In Seconds() -> (seconds since 1Jan1904=w361:timestamp)
            n138 = To Unsigned Long Integer(number=w351) -> (unsigned 32bit integer=w348:u32)
            n139 = To Unsigned Long Integer(number=w356) -> (unsigned 32bit integer=w355:u32)
            n140 = To Single Precision Float(number=w339) -> (single precision float=w338:sgl)
            n141 = while {
              shift-right: [w407] -> w359
              shift-left: w362 -> [w412]
              shift-right: [w406] -> w360
              shift-left: w363 -> [w413]
              tunnel: w361 -> [w405]
              tunnel: "Finite samples" -> [w402]
              tunnel: "N samples" -> [w404]
              shift-right: [w398] -> _
              shift-left: T9[] [] -> [w397]
              tunnel: w348 -> [w386]
              shift-right: [w393] -> _
              shift-left: T11[] [] -> [w395]
              shift-right: [w394] -> w319
              shift-left: T8[] [] -> [w396]
              tunnel: w343 -> [w392]
              tunnel: w342 -> [w391]
              tunnel: w338 -> [w390]
              tunnel: w326 -> [w379]
              shift-right: [w388] -> _
              shift-left: w328 -> [w387]
              shift-right: [w385] -> _
              shift-left: sgl[][] [] -> [w382]
              shift-right: [w384] -> _
              shift-left: u8[][] [] -> [w383]
              shift-right: [w381] -> _
              shift-left: sgl[][] [] -> [w380]
              shift-right: [w378] -> _
              shift-left: u32 1 ("x") -> [w377]
              tunnel: [FALSE] -> w318
              stop <- w399 stop-if-true
              # "stop if (((finite samples == true) && (i == Nsamples)) || (stop == true))"
              n142 = Equal?(x=w404, y=w377) -> (x = y?=w403:bool)
              n143 = VISA Read(VISA resource name=w412, byte count=u32 1, error in (no error)=w413) -> (VISA resource name out=w409:refnum<visa-resource-name>, read buffer=w410:string, error out=w408:errorcluster)  [unwired: 1 out]
              n144 = And(x=w402, y=w403) -> (x .and. y?=w400:bool)
              n145 = case shown="\"#\"" w410 {
                tunnel: w409 -> [w439 w553 w565]
                tunnel: w408 -> [w438 w552 w564]
                tunnel: [w436 w550 w565] -> w407
                tunnel: [w435 w551 w564] -> w406
                tunnel: w405 -> [w432 w547 _]
                tunnel: [w440 w546 w563] -> w398
                tunnel: w397 -> [w440 w545 w563]
                tunnel: w396 -> [w431 w542 w561]
                tunnel: w395 -> [w426 w541 w562]
                tunnel: [w430 w542 w561] -> w394
                tunnel: [w425 w541 w562] -> w393
                tunnel: w392 -> [w437 _ _]
                tunnel: w391 -> [_ w540 _]
                tunnel: w390 -> [w429 _ _]
                tunnel: [w428 FALSE ("Clock drift") FALSE ("Clock drift")] -> w389
                tunnel: w379 -> [w427 _ _]
                tunnel: [w424 w538 w559] -> w388
                tunnel: w387 -> [w423 w538 w559]
                tunnel: w386 -> [w422 _ _]
                tunnel: [w421 w536 w557] -> w385
                tunnel: w382 -> [w420 w536 w557]
                tunnel: [w419 w537 w558] -> w384
                tunnel: w383 -> [w418 w537 w558]
                tunnel: [w417 w535 w556] -> w381
                tunnel: w380 -> [w416 w535 w556]
                tunnel: [w415 w534 w555] -> w378
                tunnel: w377 -> [w414 w534 w555]
                frame "#" {
                  # "Mode case"
                  n146 = VISA Read(VISA resource name=w439, byte count=w437, error in (no error)=w438) -> (VISA resource name out=w436:refnum<visa-resource-name>, read buffer=w434:string, error out=w435:errorcluster)  [unwired: 1 out]
                  n147 = local read "Active pressure sensor constants"() -> (w433:T7[])
                  n148 = case shown="0, Default" w427 {
                    tunnel: w434 -> [w464 w507]
                    tunnel: w433 -> [w463 w506]
                    tunnel: w432 -> [w460 w503]
                    tunnel: w431 -> [w459 w508]
                    tunnel: [w458 w508] -> w430
                    tunnel: w429 -> [w457 w502]
                    tunnel: [w456 w501] -> w428
                    tunnel: w426 -> [w465 w500]
                    tunnel: [w465 w499] -> w425
                    tunnel: [w455 w494] -> w424
                    tunnel: w423 -> [w452 w490]
                    tunnel: w422 -> [w454 w491]
                    tunnel: [w450 w497] -> w421
                    tunnel: w420 -> [w449 w495]
                    tunnel: [w448 w498] -> w419
                    tunnel: w418 -> [w447 w496]
                    tunnel: [w446 w489] -> w417
                    tunnel: w416 -> [w446 w488]
                    frame 0, Default {
                      n149 = call "Process Data Buffer, Mode 0.vi"("DATA_Buffer excluding '#' [1...N]"=w464, "P constants"=w463) -> ("Pressures"=w444:sgl[], "Statuses"=w445:u8[], "dt_warn"=w461:u8)
                      n150 = Tick Count (ms)() -> (millisecond timer value=w443:u32)
                      n151 = Subtract(x=w443, y=w452) -> (x-y=w453:u32)
                      n152 = Greater Or Equal?(x=w453, y=w454) -> (x >= y?=w451:bool)
                      n153 = Bundle By Name(cluster=T8 {"Time Stamp"=timestamp(3537581686.1176577 s since 1904-01-01), "dt (us)"=0.0, "dt_warn"=0, "Pressures"=[], "Statuses"=[]} ("P data (Mode 0)"), "Time Stamp"=w460, "dt (us)"=w457, "dt_warn"=w461, "Pressures"=w444, "Statuses"=w445) -> (w441:T8)
                      n154 = Type Cast(type=FALSE ("Clock drift"), x=w461) -> (*(type *) &x=w456:bool)
                      n155 = case shown="True" w451 {
                        tunnel: [w472 w481] -> w455
                        tunnel: w452 -> [w472 _]
                        tunnel: w443 -> [_ w481]
                        tunnel: w444 -> [w471 w479]
                        tunnel: [w470 sgl[][] []] -> w450
                        tunnel: w449 -> [w469 w480]
                        tunnel: w445 -> [w468 w476]
                        tunnel: [w467 u8[][] []] -> w448
                        tunnel: w447 -> [w466 w477]
                        frame False {
                          n156 = Build Array (concatenate)(w466, w468) -> (w467:u8[][])
                          n157 = Build Array (concatenate)(w469, w471) -> (w470:sgl[][])
                        }
                        frame True {
                          n158 = Build Array (concatenate)(w477, w476) -> (→"Stale samples flag":u8[][])
                          n159 = Build Array (concatenate)(w480, w479) -> (→"Pressures time trace":sgl[][])
                        }
                      }
                      n160 = Build Array (concatenate)(w459, w441) -> (w458:T8[])
                    }
                    frame 1 {
                      n161 = call "Process Data Buffer, Mode 1.vi"("DATA_Buffer excluding '#' [1...N]"=w507, "P constants"=w506) -> ("Pressures (Pa)"=w485:sgl[], "Sensor temps (degC)"=w487:sgl[], "Statuses"=w486:u8[], "dt_warn"=w504:u8)
                      n162 = Tick Count (ms)() -> (millisecond timer value=w484:u32)
                      n163 = Subtract(x=w484, y=w490) -> (x-y=w493:u32)
                      n164 = Greater Or Equal?(x=w493, y=w491) -> (x >= y?=w492:bool)
                      n165 = Bundle By Name(cluster=T11 {"Time Stamp"=timestamp(3537581686.1176577 s since 1904-01-01), "dt (us)"=0.0, "dt_warn"=0, "Pressures"=[], "Die temps."=[], "Statuses"=[]} ("P data (Mode 1)"), "Time Stamp"=w503, "dt (us)"=w502, "dt_warn"=w504, "Pressures"=w485, "Statuses"=w486, "Die temps."=w487) -> (w482:T11)
                      n166 = Type Cast(type=FALSE ("Clock drift"), x=w504) -> (*(type *) &x=w501:bool)
                      n167 = case shown="True" w492 {
                        tunnel: [w518 w531] -> w494
                        tunnel: w490 -> [w518 _]
                        tunnel: w484 -> [_ w531]
                        tunnel: w485 -> [w517 w529]
                        tunnel: [w516 sgl[][] []] -> w497
                        tunnel: w495 -> [w515 w530]
                        tunnel: w486 -> [w514 w526]
                        tunnel: [w513 u8[][] []] -> w498
                        tunnel: w496 -> [w512 w527]
                        tunnel: [w511 sgl[][] []] -> w489
                        tunnel: w487 -> [w510 w522]
                        tunnel: w488 -> [w509 w523]
                        frame False {
                          n168 = Build Array (concatenate)(w512, w514) -> (w513:u8[][])
                          n169 = Build Array (concatenate)(w515, w517) -> (w516:sgl[][])
                          n170 = Build Array (concatenate)(w509, w510) -> (w511:sgl[][])
                        }
                        frame True {
                          n171 = Build Array (concatenate)(w527, w526) -> (w520:u8[][])
                          n172 = Build Array (concatenate)(w530, w529) -> (w519:sgl[][])
                          n173 = Build Array (concatenate)(w523, w522) -> (→"Sensor temperatures time trace (Mode \"P & T\" only)":sgl[][])
                          n174 = local write "Stale samples flag"(w520) -> ()
                          n175 = local write "Pressures time trace"(w519) -> ()
                        }
                      }
                      n176 = Build Array (concatenate)(w500, w482) -> (w499:T11[])
                    }
                  }
                  n177 = Increment(x=w414) -> (x+1=w415:u32)
                  "Samples acquired" <- w414
                }
                frame "$" {
                  n178 = local read "AccelGyro constants"() -> (w548:T3)
                  n179 = VISA Read(VISA resource name=w553, byte count=u32 29, error in (no error)=w552) -> (VISA resource name out=w550:refnum<visa-resource-name>, read buffer=w549:string, error out=w551:errorcluster)  [unwired: 1 out]
                  n180 = call "Process State Buffer.vi"("AccelGyro constants"=w548, "STATE_Buffer excluding '$' [1...30]"=w549) -> ("Inertial state values"=w543:T4, "Environmental state values"=w544:T5)
                  "Environmental state values" <- w544
                  "Inertial state values" <- w543
                  n181 = Bundle By Name(cluster=T9 {"Time Stamp"=timestamp(0 s since 1904-01-01), "dt (ms)"=0, "Environmental state values"={"Thermistor (degC)"=0.0, "Sensor temp. (degC)"=0.0, "P_atmos (Pa)"=0.0, "Rel. Humidity (%)"=0.0, "Density (kg/m^3)"=0.0, "Dew point (degC)"=0.0, "Pressure alt. (m)"=0.0, "Density alt. (m)"=0.0}, "Inertial state values"={"w_x (dps)"=0.0, "w_y (dps)"=0.0, "w_z (dps)"=0.0, "a_x (g)"=0.0, "a_y (g)"=0.0, "a_z (g)"=0.0, "Stale sample"=0, "Sensor temp. (degC)"=0.0}} ("All state values"), "Time Stamp"=w547, "dt (ms)"=w540, "Environmental state values"=w544, "Inertial state values"=w543) -> (w532:T9)
                  n182 = Build Array (concatenate)(w545, w532) -> (w546:T9[])
                }
                frame Default {
                }
              }
              "Clock drift" <- w389
              n183 = Or(x="Stop streaming", y=w400) -> (x .or. y?=w399:bool)
            }
            n184 = local read "Data rate (Hz)"() -> (w336:dbl)
            n185 = Reciprocal(x=w336) -> (1/x=w335:dbl)
            n186 = property on="Pressures time trace" class="WFChart (strict)"("XScale.Multiplier"=w335) -> ()  [unwired: 2 in, 2 out]
            n187 = property on="Sensor temperatures time trace (Mode \"P & T\" only)" class="WFChart (strict)"("XScale.Multiplier"=w335) -> ()  [unwired: 2 in, 2 out]
            n188 = local write "Streaming"(w318) -> ()
            n189 = call "Stop data stream (s).vi"("VISA resource name in"=w359, "Error In"=w360) -> ("VISA resource name out"=w357:refnum<visa-resource-name>, "Error out"=w358:errorcluster)  [unwired: 7 in]
            n190 = call "Clear buffer.vi"("Error in"=w358, "dt for timeout (ms)"=w355, "VISA resource name in"=w357) -> ("Error out"=w323:errorcluster, "VISA resource name out"=w324:refnum<visa-resource-name>)  [unwired: 3 in]
            n191 = call "Close serial port.vi"("Error in"=w323, "VISA resource name"=w324) -> ("Error out"=w320:errorcluster)  [unwired: 9 in]
          }
        }
      }
      frame "T" {
        n192 = flat-sequence {
          tunnel: w572 -> [w585]
          tunnel: w571 -> [w584]
          tunnel: [w585] -> w570
          tunnel: [w584] -> w569
          tunnel: [TRUE] -> w568
          tunnel: [w578] -> w567
          frame #0 {
            n193 = local read "Serial port"() -> (w577:refnum<visa-resource-name>)
            n194 = Divide(x=1000000.0, y="Data rate (Hz)") -> (x/y=w575:dbl)
            n195 = call "Open serial port.vi"("VISA resource name"=w577) -> ("Error out"=w581:errorcluster, "VISA resource name out"=w582:refnum<visa-resource-name>)  [unwired: 9 in]
            n196 = call "Set stream dt (T).vi"("Error In"=w581, "dt (us)"=w575, "VISA resource name in"=w582) -> ("Error out"=w580:errorcluster, "ACK"=→"ACK 2":bool, "VISA resource name out"=w579:refnum<visa-resource-name>)  [unwired: 6 in]
            n197 = call "Close serial port.vi"("Error in"=w580, "VISA resource name"=w579) -> ("Error out"=w578:errorcluster)  [unwired: 9 in]
          }
        }
      }
      frame "t" {
        n198 = flat-sequence {
          tunnel: w592 -> [w604]
          tunnel: w591 -> [w603]
          tunnel: [w604] -> w590
          tunnel: [w603] -> w589
          tunnel: [TRUE] -> w588
          tunnel: [w597] -> w587
          frame #0 {
            n199 = local read "Env. period (ms)"() -> (w594:i32)
            n200 = local read "Serial port"() -> (w595:refnum<visa-resource-name>)
            n201 = To Unsigned Long Integer(number=w594) -> (unsigned 32bit integer=w593:u32)
            n202 = call "Open serial port.vi"("VISA resource name"=w595) -> ("Error out"=w600:errorcluster, "VISA resource name out"=w601:refnum<visa-resource-name>)  [unwired: 9 in]
            n203 = call "Set state dt (t).vi"("Error In"=w600, "dt (ms)"=w593, "VISA resource name in"=w601) -> ("Error out"=w599:errorcluster, "ACK"=w596:bool, "VISA resource name out"=w598:refnum<visa-resource-name>)  [unwired: 6 in]
            n204 = call "Close serial port.vi"("Error in"=w599, "VISA resource name"=w598) -> ("Error out"=w597:errorcluster)  [unwired: 9 in]
            n205 = local write "ACK 2"(w596) -> ()
          }
        }
      }
      frame "M" {
        n206 = flat-sequence {
          tunnel: w611 -> [w623]
          tunnel: w610 -> [w622]
          tunnel: [w623] -> w609
          tunnel: [w622] -> w608
          tunnel: [TRUE] -> w607
          tunnel: [w616] -> w606
          frame #0 {
            n207 = local read "Serial port"() -> (w614:refnum<visa-resource-name>)
            n208 = call "Open serial port.vi"("VISA resource name"=w614) -> ("Error out"=w619:errorcluster, "VISA resource name out"=w620:refnum<visa-resource-name>)  [unwired: 9 in]
            n209 = call "Set mode (M).vi"("Error In"=w619, "Mode"="Data mode", "VISA resource name in"=w620) -> ("Error out"=w618:errorcluster, "ACK"=w615:bool, "L_data"=→"L_data (bytes)":u16, "VISA resource name out"=w617:refnum<visa-resource-name>)  [unwired: 5 in]
            n210 = call "Close serial port.vi"("Error in"=w618, "VISA resource name"=w617) -> ("Error out"=w616:errorcluster)  [unwired: 9 in]
            n211 = local write "ACK 2"(w615) -> ()
          }
        }
      }
      frame "O" {
        n212 = flat-sequence {
          tunnel: w630 -> [w642]
          tunnel: w629 -> [w641]
          tunnel: [w642] -> w628
          tunnel: [w641] -> w627
          tunnel: [TRUE] -> w626
          tunnel: [w635] -> w625
          frame #0 {
            n213 = local read "Serial port"() -> (w634:refnum<visa-resource-name>)
            n214 = call "Open serial port.vi"("VISA resource name"=w634) -> ("Error out"=w638:errorcluster, "VISA resource name out"=w639:refnum<visa-resource-name>)  [unwired: 9 in]
            n215 = call "Override maxSensorNum (O).vi"("Error In"=w638, "Max. number of sensors"="Max. num. sensors (override)", "VISA resource name in"=w639) -> ("Error out"=w637:errorcluster, "ACK"=→"ACK 3":bool, "L_data"=w631:u16, "VISA resource name out"=w636:refnum<visa-resource-name>)  [unwired: 5 in]
            n216 = local write "L_data (bytes)"(w631) -> ()
            n217 = call "Close serial port.vi"("Error in"=w637, "VISA resource name"=w636) -> ("Error out"=w635:errorcluster)  [unwired: 9 in]
          }
        }
      }
      frame "G" {
        n218 = flat-sequence {
          tunnel: w649 -> [w665]
          tunnel: w648 -> [w664]
          tunnel: [w665] -> w647
          tunnel: [w664] -> w646
          tunnel: [TRUE] -> w645
          tunnel: [w658] -> w644
          frame #0 {
            n219 = local read "Serial port"() -> (w657:refnum<visa-resource-name>)
            n220 = call "Open serial port.vi"("VISA resource name"=w657) -> ("Error out"=w661:errorcluster, "VISA resource name out"=w662:refnum<visa-resource-name>)  [unwired: 9 in]
            n221 = call "Get status bits 1 (G).vi"("VISA resource name in"=w662, "Error In"=w661) -> ("nFaults"=w654:u8, "nSensors"=w653:u8, "nCards"=w652:u8, "PowerState"=w651:bool, "VISA resource name out"=w659:refnum<visa-resource-name>, "ACK"=→"ACK 5":bool, "Error out"=w660:errorcluster)  [unwired: 11 in]
            n222 = local read "System status"() -> (w650:T6)
            n223 = call "Close serial port.vi"("Error in"=w660, "VISA resource name"=w659) -> ("Error out"=w658:errorcluster)  [unwired: 9 in]
            n224 = Bundle By Name(cluster=w650, "Main power"=w651, "Occupied slots"=w652, "Active sensors"=w653, "Faulty sensors"=w654) -> (→"System status":T6)
          }
        }
      }
      frame "g" {
        n225 = flat-sequence {
          tunnel: w672 -> [w693]
          tunnel: w671 -> [w692]
          tunnel: [w693] -> w670
          tunnel: [w692] -> w669
          tunnel: [TRUE] -> w668
          tunnel: [w686] -> w667
          frame #0 {
            w675 = T12."Disabled and Grayed Out" ("Disabled")
            w674 = T12."Enabled" ("Disabled")
            n226 = local read "Serial port"() -> (w685:refnum<visa-resource-name>)
            n227 = call "Open serial port.vi"("VISA resource name"=w685) -> ("Error out"=w689:errorcluster, "VISA resource name out"=w690:refnum<visa-resource-name>)  [unwired: 9 in]
            n228 = call "Get status bits 2 (g).vi"("VISA resource name in"=w690, "Error In"=w689) -> ("Mode"=w684:u8, "Therm_ok"=w676:bool, "BMI160_ok"=w680:bool, "BME280_ok"=w678:bool, "VISA resource name out"=w687:refnum<visa-resource-name>, "ACK"=w682:bool, "Error out"=w688:errorcluster)  [unwired: 11 in]
            n229 = Select(t=w674, s=w676, f=w675) -> (s? t:f=w679:T12)
            n230 = Select(t=w674, s=w678, f=w675) -> (s? t:f=w677:T12)
            n231 = stacked-sequence {
              tunnel: w679 -> [_ w695]
              tunnel: w677 -> [w694 _]
              tunnel: w676 -> [_ w696]
              frame #0 {
                n232 = property on="Environmental state values" class="Clust (strict)"("DisabledEnum"=w694) -> ()  [unwired: 2 in, 2 out]
                n233 = property on="Density (kg/m^3)" class="DigNum (strict)"("DisabledEnum"=w694) -> ()  [unwired: 2 in, 2 out]
                n234 = property on="Dew point (degC)" class="DigNum (strict)"("DisabledEnum"=w694) -> ()  [unwired: 2 in, 2 out]
                n235 = property on="Density alt. (m)" class="DigNum (strict)"("DisabledEnum"=w694) -> ()  [unwired: 2 in, 2 out]
              }
              frame #1 {
                n236 = case shown="False" w696 {
                  tunnel: w695 -> [w697 _]
                  frame False {
                    n237 = property on="Density (kg/m^3)" class="DigNum (strict)"("DisabledEnum"=w697) -> ()  [unwired: 2 in, 2 out]
                    n238 = property on="Dew point (degC)" class="DigNum (strict)"("DisabledEnum"=w697) -> ()  [unwired: 2 in, 2 out]
                    n239 = property on="Density alt. (m)" class="DigNum (strict)"("DisabledEnum"=w697) -> ()  [unwired: 2 in, 2 out]
                  }
                  frame True {
                  }
                }
                n240 = property on="Thermistor (degC)" class="DigNum (strict)"("DisabledEnum"=w695) -> ()  [unwired: 2 in, 2 out]
              }
            }
            n241 = local read "System status"() -> (w681:T6)
            n242 = call "Close serial port.vi"("Error in"=w688, "VISA resource name"=w687) -> ("Error out"=w686:errorcluster)  [unwired: 9 in]
            n243 = local write "ACK 5"(w682) -> ()
            n244 = Select(t=w674, s=w680, f=w675) -> (s? t:f=w673:T12)
            n245 = Bundle By Name(cluster=w681, "Env. sensor"=w678, "Inertial sensor"=w680, "Thermistor"=w676, "Mode"=w684) -> (w683:T6)
            n246 = property on="Inertial state values" class="Clust (strict)"("DisabledEnum"=w673) -> ()  [unwired: 2 in, 2 out]
            n247 = property on="AccelGyro constants" class="Clust (strict)"("DisabledEnum"=w673) -> ()  [unwired: 2 in, 2 out]
            n248 = property on="Accel. range (g)" class="Ring (strict)"("DisabledEnum"=w673) -> ()  [unwired: 2 in, 2 out]
            n249 = property on="Accel. rate (Hz)" class="Ring (strict)"("DisabledEnum"=w673) -> ()  [unwired: 2 in, 2 out]
            n250 = property on="Gyro. range (dps)" class="Ring (strict)"("DisabledEnum"=w673) -> ()  [unwired: 2 in, 2 out]
            n251 = property on="Gyro. rate (Hz)" class="Ring (strict)"("DisabledEnum"=w673) -> ()  [unwired: 2 in, 2 out]
            n252 = property on="ACK 8" class="Bool (strict)"("DisabledEnum"=w673) -> ()  [unwired: 2 in, 2 out]
            n253 = local write "System status"(w683) -> ()
          }
        }
      }
      frame "F" {
        n254 = flat-sequence {
          tunnel: w704 -> [w714]
          tunnel: w703 -> [w713]
          tunnel: [w714] -> w702
          tunnel: [w713] -> w701
          tunnel: [TRUE] -> w700
          tunnel: [w707] -> w699
          frame #0 {
            n255 = local read "Serial port"() -> (w706:refnum<visa-resource-name>)
            n256 = call "Open serial port.vi"("VISA resource name"=w706) -> ("Error out"=w710:errorcluster, "VISA resource name out"=w711:refnum<visa-resource-name>)  [unwired: 9 in]
            n257 = call "Collate faulty sensor indices.vi"("Error In"=w710, "VISA resource name in"=w711) -> ("Error out"=w709:errorcluster, "Faulty sensor indices"=→"Faulty sensors":i32[], "VISA resource name out"=w708:refnum<visa-resource-name>)  [unwired: 7 in]
            n258 = call "Close serial port.vi"("Error in"=w709, "VISA resource name"=w708) -> ("Error out"=w707:errorcluster)  [unwired: 9 in]
          }
        }
      }
      frame "A" {
        n259 = flat-sequence {
          tunnel: w721 -> [w731]
          tunnel: w720 -> [w730]
          tunnel: [w731] -> w719
          tunnel: [w730] -> w718
          tunnel: [TRUE] -> w717
          tunnel: [w724] -> w716
          frame #0 {
            n260 = local read "Serial port"() -> (w723:refnum<visa-resource-name>)
            n261 = call "Open serial port.vi"("VISA resource name"=w723) -> ("Error out"=w727:errorcluster, "VISA resource name out"=w728:refnum<visa-resource-name>)  [unwired: 9 in]
            n262 = call "Collate active sensor indices.vi"("Error In"=w727, "VISA resource name in"=w728) -> ("Error out"=w726:errorcluster, "Active sensor indices"=→"Active sensors":i32[], "VISA resource name out"=w725:refnum<visa-resource-name>)  [unwired: 7 in]
            n263 = call "Close serial port.vi"("Error in"=w726, "VISA resource name"=w725) -> ("Error out"=w724:errorcluster)  [unwired: 9 in]
          }
        }
      }
      frame "C" {
        n264 = flat-sequence {
          tunnel: w738 -> [w756]
          tunnel: w737 -> [w755]
          tunnel: [w756] -> w736
          tunnel: [w755] -> w735
          tunnel: [TRUE] -> w734
          tunnel: [w749] -> w733
          frame #0 {
            n265 = local read "Serial port"() -> (w748:refnum<visa-resource-name>)
            n266 = call "Open serial port.vi"("VISA resource name"=w748) -> ("Error out"=w752:errorcluster, "VISA resource name out"=w753:refnum<visa-resource-name>)  [unwired: 9 in]
            n267 = call "Configure BMI160 (C).vi"("VISA resource name in"=w753, "Accel. range (g)"="Accel. range (g)", "Accel. rate (Hz)"="Accel. rate (Hz)", "Gyro. range (dps)"="Gyro. range (dps)", "Gyro. rate (Hz)"="Gyro. rate (Hz)", "Error In"=w752) -> ("VISA resource name out"=w750:refnum<visa-resource-name>, "ACK ok"=→"ACK 4":bool, "Error out"=w751:errorcluster)  [unwired: 11 in]
            n268 = case shown="0, Default" "Accel. range (g)" {
              tunnel: [sgl 2.0 ("accRange") sgl 4.0 ("accRange") sgl 8.0 ("accRange") sgl 16.0 ("accRange")] -> w742
              frame 0, Default {
              }
              frame 1 {
              }
              frame 2 {
              }
              frame 3 {
              }
            }
            n269 = case shown="0, Default" "Gyro. range (dps)" {
              tunnel: [sgl 125.0 ("accRange") sgl 250.0 ("accRange") sgl 500.0 ("accRange") sgl 1000.0 ("accRange") sgl 2000.0 ("accRange")] -> w740
              frame 0, Default {
              }
              frame 1 {
              }
              frame 2 {
              }
              frame 3 {
              }
              frame 4 {
              }
            }
            n270 = call "Close serial port.vi"("Error in"=w751, "VISA resource name"=w750) -> ("Error out"=w749:errorcluster)  [unwired: 9 in]
            n271 = local read "AccelGyro constants"() -> (w739:T3)
            n272 = Bundle By Name(cluster=w739, "accRange"=w742, "gyrRange"=w740) -> (w744:T3)
            n273 = local write "AccelGyro constants"(w744) -> ()
          }
        }
      }
      frame "Z" {
        n274 = flat-sequence {
          tunnel: w772 -> [w782]
          tunnel: w771 -> [w781]
          tunnel: [w782] -> w770
          tunnel: [w781] -> w769
          tunnel: [TRUE] -> w768
          tunnel: [w775] -> w767
          frame #0 {
            n275 = local read "Serial port"() -> (w774:refnum<visa-resource-name>)
            n276 = call "Open serial port.vi"("VISA resource name"=w774) -> ("Error out"=w778:errorcluster, "VISA resource name out"=w779:refnum<visa-resource-name>)  [unwired: 9 in]
            n277 = call "Get Serial Number (Z).vi"("VISA resource name in"=w779, "Error In"=w778) -> ("VISA resource name out"=w776:refnum<visa-resource-name>, "Serial Number"=→"Serial no.":u16, "Error out"=w777:errorcluster)  [unwired: 5 in, 1 out]
            n278 = call "Close serial port.vi"("Error in"=w777, "VISA resource name"=w776) -> ("Error out"=w775:errorcluster)  [unwired: 9 in]
          }
        }
      }
      frame "D" {
        n279 = flat-sequence {
          tunnel: w790 -> [w812]
          tunnel: w789 -> [w811]
          tunnel: [w812] -> w788
          tunnel: [w811] -> w787
          tunnel: [TRUE] -> w786
          tunnel: [w791] -> w785
          tunnel: [w796] -> w784
          tunnel: w783 -> [w797]
          frame #0 {
            # "write after interval has passed, else append"
            n280 = local read "AccelGyro constants"() -> (w801:T3)
            n281 = local read "Serial port"() -> (w809:refnum<visa-resource-name>)
            n282 = call "Open serial port.vi"("VISA resource name"=w809) -> ("Error out"=w807:errorcluster, "VISA resource name out"=w808:refnum<visa-resource-name>)  [unwired: 9 in]
            n283 = call "Get Env data (oneshot) (D).vi"("VISA resource name in"=w808, "Error In"=w807) -> ("VISA resource name out"=w805:refnum<visa-resource-name>, "STATE_Buffer"=w804:string, "ACK"=→"ACK 6":bool, "Error out"=w806:errorcluster)  [unwired: 5 in]
            n284 = local read "Env. period (ms)"() -> (w794:i32)
            n285 = Get Date/Time In Seconds() -> (seconds since 1Jan1904=w792:timestamp)
            n286 = call "Close serial port.vi"("Error in"=w806, "VISA resource name"=w805) -> ("Error out"=w791:errorcluster)  [unwired: 9 in]
            n287 = String Subset(string=w804, offset (0)=1) -> (substring=w803:string)  [unwired: 1 in]
            n288 = call "Process State Buffer.vi"("AccelGyro constants"=w801, "STATE_Buffer excluding '$' [1...30]"=w803) -> ("Inertial state values"=w798:T4, "Environmental state values"=w799:T5)
            n289 = Bundle By Name(cluster=T9 {"Time Stamp"=timestamp(0 s since 1904-01-01), "dt (ms)"=0, "Environmental state values"={"Thermistor (degC)"=0.0, "Sensor temp. (degC)"=0.0, "P_atmos (Pa)"=0.0, "Rel. Humidity (%)"=0.0, "Density (kg/m^3)"=0.0, "Dew point (degC)"=0.0, "Pressure alt. (m)"=0.0, "Density alt. (m)"=0.0}, "Inertial state values"={"w_x (dps)"=0.0, "w_y (dps)"=0.0, "w_z (dps)"=0.0, "a_x (g)"=0.0, "a_y (g)"=0.0, "a_z (g)"=0.0, "Stale sample"=0, "Sensor temp. (degC)"=0.0}} ("All state values"), "Time Stamp"=w792, "dt (ms)"=w794, "Environmental state values"=w799, "Inertial state values"=w798) -> (w793:T9)
            n290 = local write "Environmental state values"(w799) -> ()
            n291 = local write "Inertial state values"(w798) -> ()
            n292 = Build Array (concatenate)(w797, w793) -> (w796:T9[])
          }
        }
      }
      frame "accgyr_consts" {
        n293 = flat-sequence {
          tunnel: w819 -> [w839]
          tunnel: w818 -> [w838]
          tunnel: [w839] -> w817
          tunnel: [w838] -> w816
          tunnel: [TRUE] -> w815
          tunnel: [w836] -> w814
          frame #0 {
            n294 = local read "Serial port"() -> (w835:refnum<visa-resource-name>)
            n295 = call "Open serial port.vi"("VISA resource name"=w835) -> ("Error out"=w833:errorcluster, "VISA resource name out"=w834:refnum<visa-resource-name>)  [unwired: 9 in]
            n296 = call "Get AccelGyro constants (MCU EEPROM).vi"("VISA resource name in"=w834, "Error In"=w833) -> ("VISA resource name out"=w831:refnum<visa-resource-name>, "AccelGyro constants"=w828:T3, "ACK"=→"ACK 8":bool, "Error out"=w832:errorcluster)  [unwired: 5 in]
            n297 = Unbundle By Name(w828) -> ("gx offset"=w827:sgl, "gy offset"=w826:sgl, "gz offset"=w825:sgl, "ax offset"=w824:sgl, "ay offset"=w823:sgl, "az offset"=w822:sgl, "axyz scale"=w821:sgl)
            n298 = call "Close serial port.vi"("Error in"=w832, "VISA resource name"=w831) -> ("Error out"=w836:errorcluster)  [unwired: 9 in]
            n299 = Bundle By Name(cluster=T3 {"gyrRange"=125.0, "accRange"=2.0, "gx offset"=0.0, "gy offset"=0.0, "gz offset"=0.0, "ax offset"=0.0, "ay offset"=0.0, "az offset"=0.0, "axyz scale"=1.0} ("AccelGyro constants"), "gx offset"=w827, "gy offset"=w826, "gz offset"=w825, "ax offset"=w824, "ay offset"=w823, "az offset"=w822, "axyz scale"=w821) -> (→"AccelGyro constants":T3)
          }
        }
      }
      frame "EEPROM_Pconsts" {
        n300 = flat-sequence {
          tunnel: w846 -> [w862]
          tunnel: w845 -> [w861]
          tunnel: [w862] -> w844
          tunnel: [w861] -> w843
          tunnel: [TRUE] -> w842
          tunnel: [w859] -> w841
          frame #0 {
            # "Must only run this case after running \"P\", \"G\", \"A\""
            n301 = local read "System status"() -> (w851:T6)
            n302 = Unbundle By Name(w851) -> ("Occupied slots"=w850:u8)
            n303 = local read "Serial port"() -> (w858:refnum<visa-resource-name>)
            n304 = To Long Integer(number=w850) -> (32bit integer=w849:i32)
            n305 = call "Open serial port.vi"("VISA resource name"=w858) -> ("Error out"=w856:errorcluster, "VISA resource name out"=w857:refnum<visa-resource-name>)  [unwired: 9 in]
            n306 = local read "Active sensors"() -> (w853:i32[])
            n307 = call "Concatenate all slot EEPROM arrays.vi"("Error In"=w856, "N slots occupied"=w849, "VISA resource name in"=w857) -> ("Error out"=w855:errorcluster, "ACK (all)"=→"ACK 7":bool, "All slot EEPROM values"=w848:T13[], "VISA resource name out"=w854:refnum<visa-resource-name>)  [unwired: 5 in]
            n308 = call "Populate pressure constants array.vi"("Occupied slot EEPROM values"=w848, "Active sensor indices"=w853) -> ("Active pressure sensor constants"=→"Active pressure sensor constants":T7[])
            n309 = call "Close serial port.vi"("Error in"=w855, "VISA resource name"=w854) -> ("Error out"=w859:errorcluster)  [unwired: 9 in]
          }
        }
      }
      frame "Exit", Default {
      }
    }
    n310 = Get Queue Status(queue=w239, return elements? (F)=FALSE, error in (no error)=w238) -> (queue out=w233:refnum<queue>, error out=w236:errorcluster, # elements in queue=w235:i32)  [unwired: 5 out]
    n311 = call <vilib>:"Clear Errors.vi"("error in (no error)"=w241, "specific error code to clear (0: all)"=1073676294) -> ("error out"=w240:errorcluster)  [unwired: 4 in, 1 out]
    "Error out" <- w240
    n312 = Equal To 0?(x=w235) -> (x = 0?=w234:bool)
  }
  "P data (mode 0)" <- w3
  n313 = Release Queue(queue=w9, error in (no error)=w15) -> (error out=w10:errorcluster)  [unwired: 1 in, 2 out]
  n314 = Merge Errors(w10, w11) -> (w12:errorcluster)
  n315 = local write "Error out"(w12) -> ()
